vi "prepare_and_upload.vi"() -> ()   [LabVIEW 2016]
uses:
  <userlib>/LevyLab/Graph Utilities/graph_utilities.lvclass
  <userlib>/LevyLab/LV to ITX/Data/Data.lvclass
  <userlib>/LevyLab/postgreSQL-timescaleDB/Data.S3/Data.S3.lvclass
  <userlib>/LevyLab/postgreSQL-timescaleDB/Data.PG/Data.PGSQL.lvclass
  <userlib>/LevyLab/Graph Utilities/graph_utilities.lvclass/graph_utilities.ctl
  <userlib>/LevyLab/LV to ITX/Data/Data.lvclass/Data.ctl
  subvi/operationQueue/fft/fft_typedef.ctl
  subvi/operationQueue/derivative/derivative_typedef.ctl
  <userlib>/LevyLab/LV to ITX/Data/Typedefs/File Type--enum.ctl
  <userlib>/_OpenG.lib/file/file.llb/File Exists - Scalar__ogtk.vi
  <userlib>/_OpenG.lib/dictionary/dictionary.llb/Dictionary Update (by scalar value)__ogtk.vi
  <userlib>/LevyLab/XY Utilities/subVIs/Derivative (multiple).vi
  <userlib>/_OpenG.lib/file/file.llb/Build Path - File Names Array__ogtk.vi
  <userlib>/LevyLab/XY Utilities/xy_utilities.lvlib
  <userlib>/LevyLab/LV to ITX/Macros/Conversion.lvclass
panel:
  out "selected.local path":path
  out "generated tdms file path":path
  out "Intensity Graph":dbl[][](graph)
  out "Wavenames":string[](array[string])
  out "Notes":string
  out "Vertical Linecut":cluster{"Array":dbl[], "A x Vector":dbl[]}[](graph) caption="XY Graph"
  out "Horizontal Linecut":cluster{"Array":dbl[], "A x Vector":dbl[]}[](graph) caption="XY Graph"
  in  "# std deviations for\nhistogram width":dbl(slide)=1.4340101522842639 scale=0.0..5.0
  out "Histogram Graph":T1(graph)={"X Values"=[-4.260453721936876e-06, -4.186170219584622e-06, -4.111886717232367e-06, -4.037603214880112e-06, -3.9633197125278575e-06, -3.889036210175604e-06, -3.814752707823349e-06, -3.7404692054710943e-06, -3.6661857031188396e-06, -3.591902200766585e-06, -3.5176186984143303e-06, -3.4433351960620756e-06, -3.369051693709821e-06, -3.294768191357566e-06, -3.2204846890053115e-06, -3.1462011866530572e-06, -3.0719176843008025e-06, -2.9976341819485483e-06, -2.9233506795962936e-06, -2.849067177244039e-06, -2.774783674891784e-06, -2.7005001725395295e-06, -2.626216670187275e-06, -2.55193316783502e-06, -2.4776496654827654e-06, -2.4033661631305107e-06, -2.3290826607782565e-06, -2.2547991584260018e-06, -2.180515656073747e-06, -2.106232153721493e-06, -2.031948651369238e-06, -1.9576651490169834e-06, -1.8833816466647288e-06, -1.809098144312474e-06, -1.7348146419602196e-06, -1.6605311396079651e-06, -1.5862476372557104e-06, -1.5119641349034557e-06, -1.437680632551201e-06, -1.3633971301989466e-06, -1.289113627846692e-06, -1.2148301254944374e-06, -1.1405466231421827e-06, -1.066263120789928e-06, -9.919796184376733e-07, -9.176961160854188e-07, -8.434126137331644e-07, -7.691291113809097e-07, -6.94845609028655e-07, -6.205621066764003e-07, -5.462786043241458e-07, -4.7199510197189133e-07, -3.9771159961963664e-07, -3.2342809726738195e-07, -2.4914459491512726e-07, -1.7486109256287257e-07, -1.0057759021061788e-07, -2.6294087858363186e-08, 4.798941449389108e-08, 1.2227291684614535e-07, 1.9655641919840004e-07, 2.7083992155065473e-07, 3.451234239029094e-07, 4.194069262551641e-07, 4.936904286074188e-07, 5.679739309596735e-07, 6.422574333119282e-07, 7.165409356641829e-07, 7.908244380164376e-07, 8.651079403686918e-07, 9.393914427209461e-07, 1.0136749450732008e-06, 1.0879584474254555e-06, 1.1622419497777102e-06, 1.2365254521299649e-06, 1.3108089544822195e-06, 1.3850924568344742e-06, 1.459375959186729e-06, 1.5336594615389836e-06, 1.6079429638912379e-06, 1.6822264662434922e-06, 1.7565099685957468e-06, 1.8307934709480015e-06, 1.9050769733002562e-06, 1.979360475652511e-06, 2.0536439780047656e-06, 2.1279274803570203e-06, 2.202210982709275e-06, 2.2764944850615297e-06, 2.3507779874137844e-06, 2.4250614897660386e-06, 2.499344992118293e-06, 2.5736284944705476e-06, 2.6479119968228023e-06, 2.722195499175057e-06, 2.7964790015273117e-06, 2.8707625038795664e-06, 2.945046006231821e-06, 3.0193295085840757e-06, 3.09361301093633e-06], "Histogram: h(x)"=[55, 64, 64, 55, 89, 72, 77, 95, 93, 93, 89, 83, 103, 107, 94, 103, 104, 123, 108, 131, 122, 143, 132, 148, 168, 174, 204, 248, 183, 187, 243, 200, 217, 226, 238, 254, 185, 182, 212, 219, 221, 318, 385, 545, 593, 736, 735, 784, 778, 858, 957, 1241, 1705, 2411, 3715, 13259, 21719, 20305, 20447, 22279, 10136, 3576, 2142, 1564, 1112, 936, 844, 776, 734, 696, 601, 535, 390, 337, 334, 301, 271, 341, 294, 279, 254, 216, 170, 148, 122, 140, 100, 114, 127, 147, 102, 114, 129, 135, 110, 105, 90, 91, 93, 96]}
  in  "menu select":T2(tab)
  in  "Upload TDMS button":bool
  in  "View before uploading?":bool
  out "Converting Indicator":bool
  out "Uploading Indicator":bool
  in  "Populate Local Tree":bool
  in  "Local Tree":string(tree)
  in  "Populate Remote Tree":bool
  in  "local data directory":path=path "C:/bigdata/PPMS2/SA03008N.20190801/031_sg1_-1'1''5m_3AC=500m_bg=-14" caption="Path"
  out "Visualizing Indicator":bool
  out "TDMS load (ms)":u32
  out "data dimensions":i32[](array[numeric])
  in  "Remote Tree":string(tree)
  in  "path to aws credentials":path=path "C:/Users/phil/.aws/credentials"
  in  "aws bucket":string="levylab-data"
  out "generate TDMS (ms)":u32
  out "S3 upload (ms)":u32
  in  "connection info":T3
  in  "Operation Config":enum32{"derivative", "fft"}(tab)
  in  "derivative":T4={"derivative"="derivative", "Interval"=2.0, "Interval Units"=enum."Points", "Type"=enum."dy/dx vs x"}
  in  "Add Op":bool
  in  "Operations List":i32(listbox)
  in  "update":bool
  out "slicing\ntime":i32
  out "updating":bool
  in  "auto\nupdate":bool
  in  "trash can":i32(listbox)
  in  "OK":bool
  # "temporary things:"
  # "4"
  # "7"
  # "10"
  # "12"
  # "14"
  # "Settings"
  # "17"
  # "e.g. SA03008N.20190801"
  # "DON'T DOUBLE CLICK BIG FOLDERS"
  # ":)"
  # "not yet implemented"
  # "no settings"
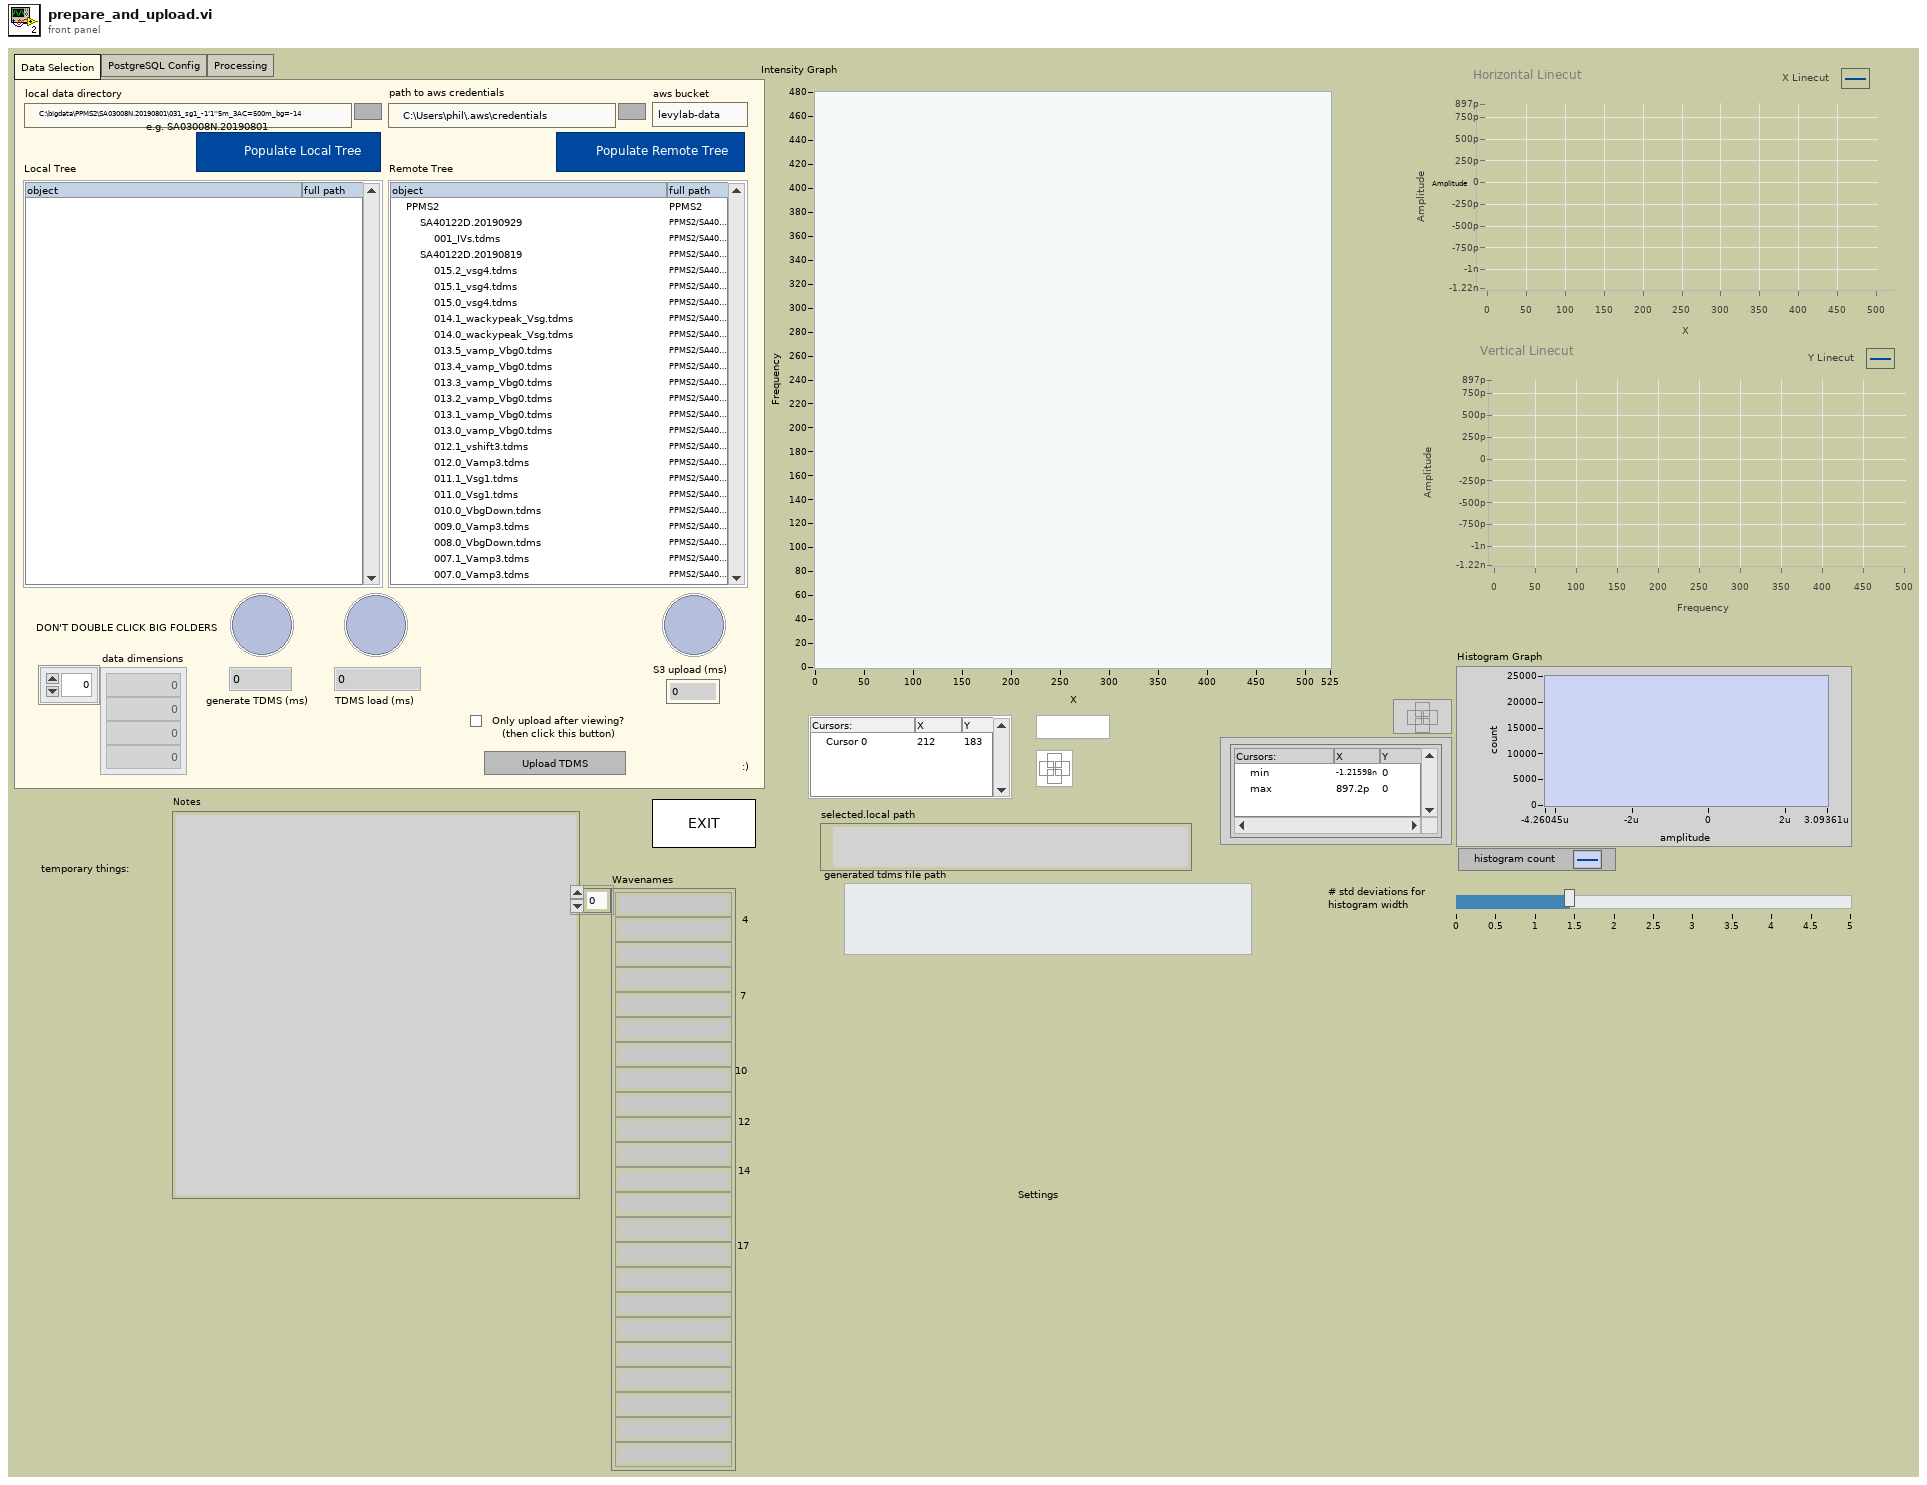
[diagram p1: front panel]
types:
  T1 = cluster{"X Values":dbl[], "Histogram: h(x)":i32[]}
  T2 = enum32{"Data Selection", "PostgreSQL Config", "Processing"}
  T3 = cluster{"host":string, "port":string, "user":string, "dbname":string, "password":string}
  T4 = cluster{"derivative":string, "Interval":dbl, "Interval Units":enum16{"Points", "Data"}, "Type":enum16{"dy/dx vs x", "dx/dy vs y"}}
  T5 = enum32{"Invalid", "Standard", "Closed", "Hidden", "Minimized", "Maximized"}
  T6 = enum32{"invalid app kind", "Development System", "Run Time System", "Student Edition", "Embedded LabVIEW", "Evaluation", "Custom"}
  T7 = typedef "fft_typedef.ctl" = cluster{"fft":string}
  T8 = typedef "derivative_typedef.ctl" = cluster{"derivative":string, "Interval":dbl, "Interval Units":enum16{"Points", "Data"}, "Type":enum16{"dy/dx vs x", "dx/dy vs y"}}
  T9 = typedef "Data.lvclass/File Type--enum.ctl" = enum16{"DAT", "ITX", "TDMS", "VI"}
  T10 = typedef "Dictionary Object RefNum__ogtk.ctl" = refnum<k1>
  T11 = cluster{"Core":cluster{"Current VI Reference":refnum<vi>, "Close Panel on Exit?":bool}, "active XY data":cluster{"All expt data":dbl[], "All expt data":dbl[]}[], "local data directory":path, "Data Save":refnum<class "Data.lvclass">, "graphs":refnum<class "graph_utilities.lvclass">[], "dictionary out":T10, "Operations List":refnum<vi>, "operations performed":string[], "Histogram Data":cluster{"X Values":dbl[], "Histogram: h(x)":i32[]}, "Histogram Graph":refnum<vi>, "wavenames":string[], "Data.S3":refnum<class "Data.S3.lvclass">, "data dimensions":i32[], "Data.PG in":refnum<class "Data.PGSQL.lvclass">, "selected":cluster{"local path":path, "\\ remote path":string, "/ remote path":string}, "generated tdms":path, "uploaded remote path":string}
  T12 = cluster{"local path":path, "\\ remote path":string, "/ remote path":string}
  T13 = cluster{"All expt data":dbl[], "All expt data":dbl[]}[]
  T14 = cluster{"Current VI Reference":refnum<vi>, "Close Panel on Exit?":bool}
  T15 = typedef "Data.lvclass/Dictionary--cluster.ctl" = cluster{"key":string, "value":variant}
  T16 = cluster{"concatenated string":string, "derivative":cluster{"derivative":string, "Interval":dbl, "Interval Units":enum16{"Points", "Data"}, "Type":enum16{"dy/dx vs x", "dx/dy vs y"}}}
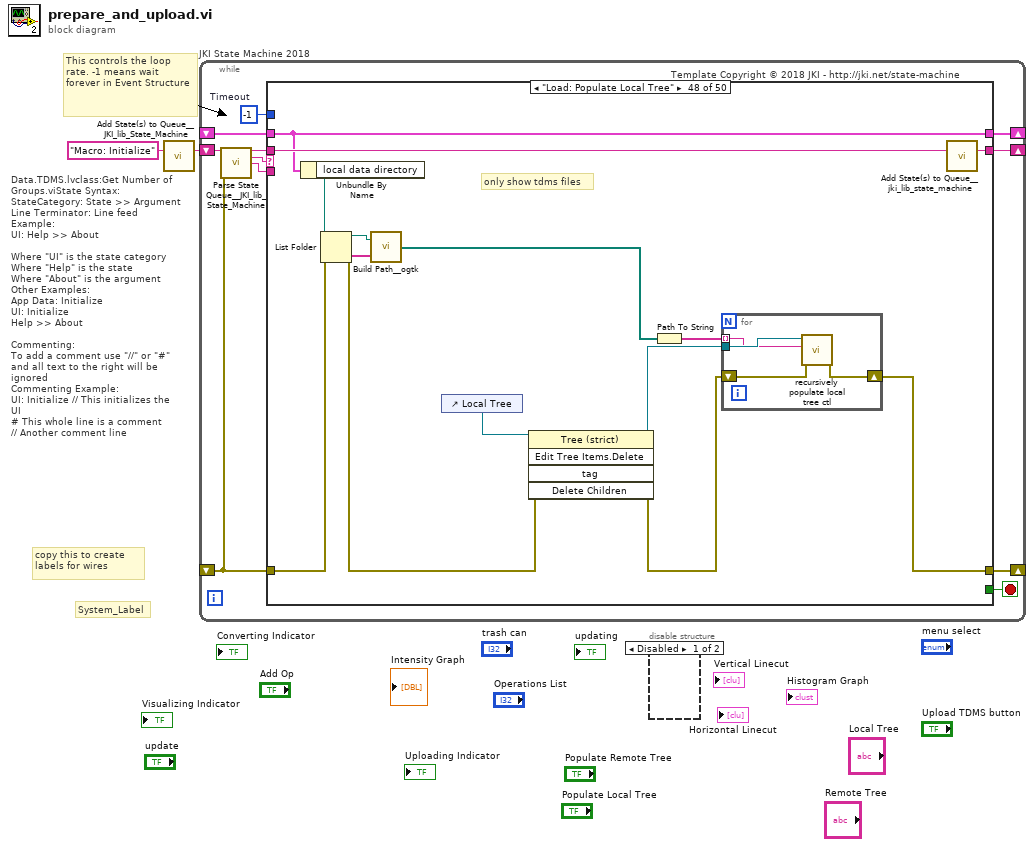
[diagram p0: block diagram]
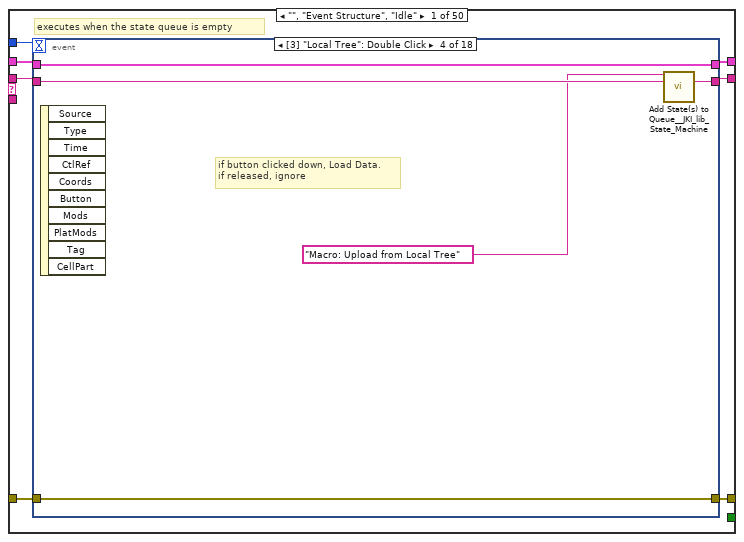
[diagram p3: hidden frame]
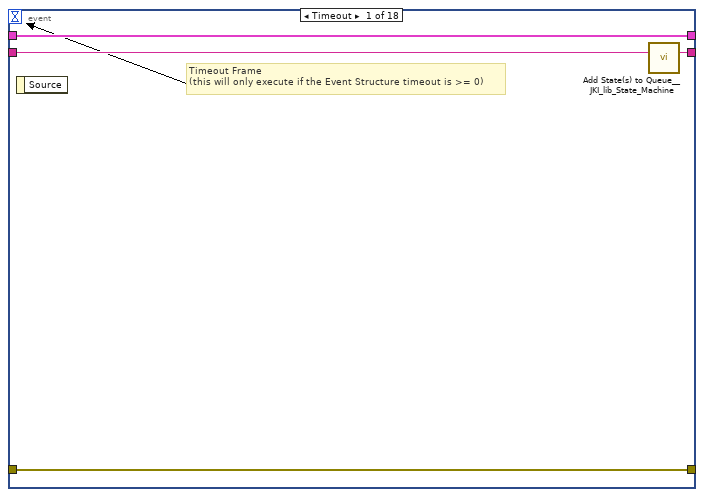
[diagram p4: hidden frame]
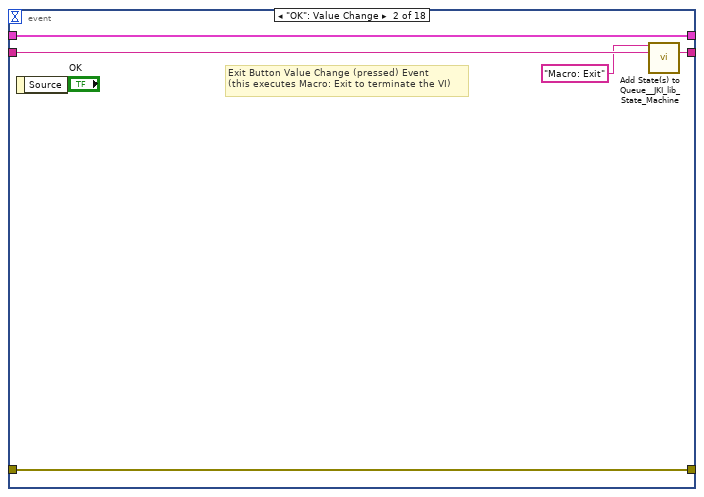
[diagram p5: hidden frame]
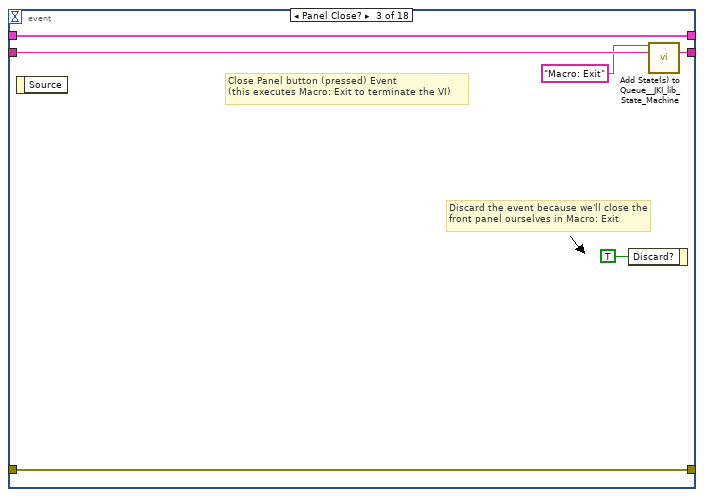
[diagram p6: hidden frame]
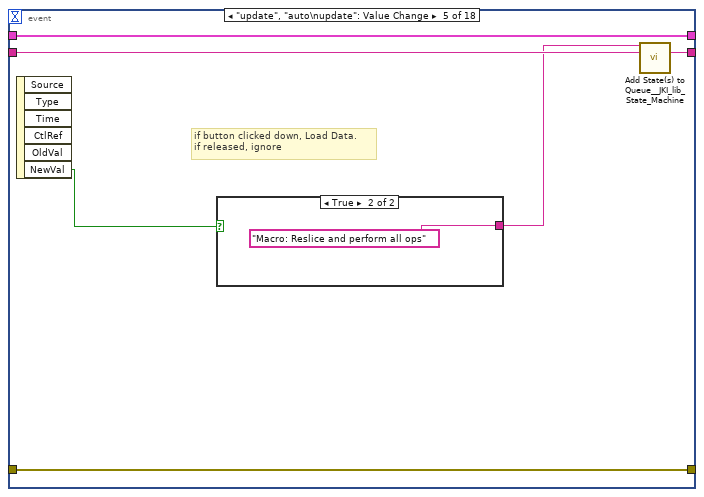
[diagram p7: hidden frame]
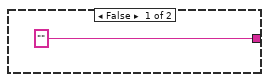
[diagram p8: hidden frame]
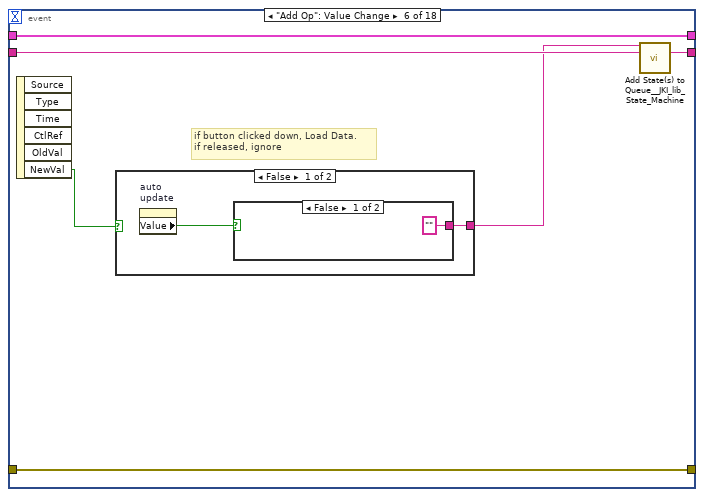
[diagram p9: hidden frame]
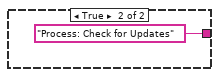
[diagram p10: hidden frame]
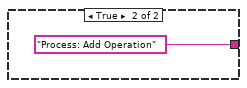
[diagram p11: hidden frame]
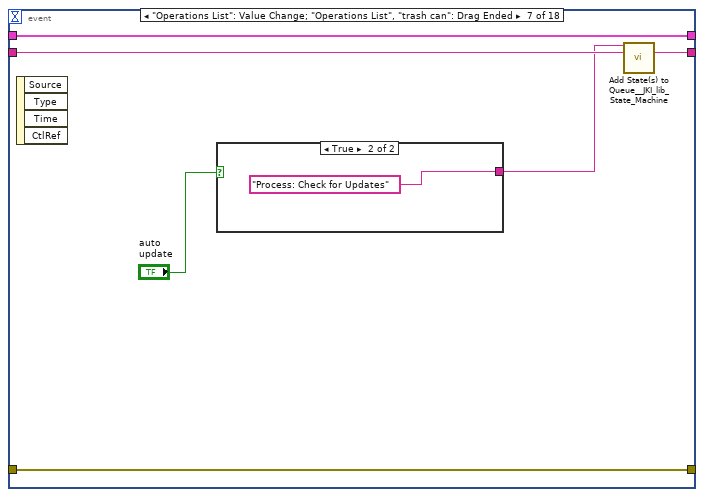
[diagram p12: hidden frame]
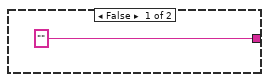
[diagram p13: hidden frame]
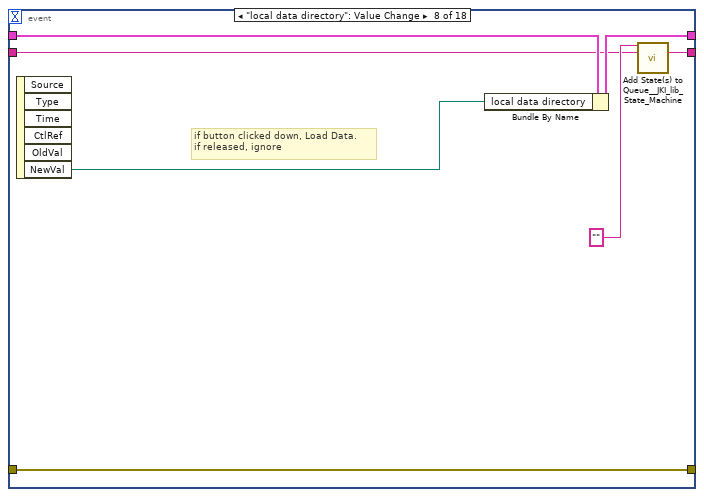
[diagram p14: hidden frame]
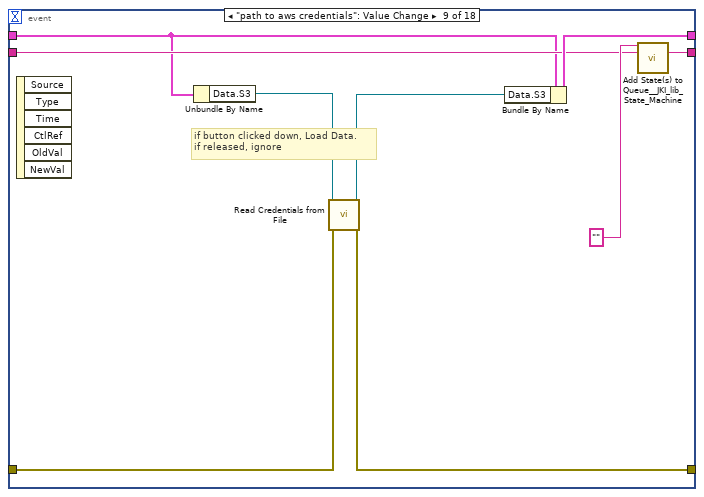
[diagram p15: hidden frame]
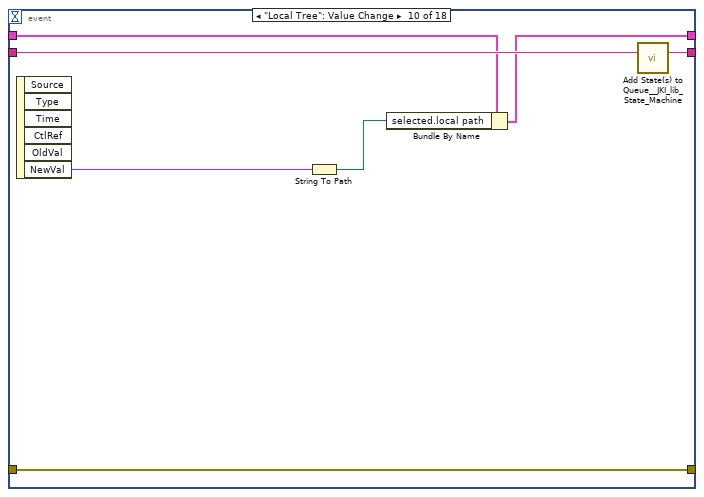
[diagram p16: hidden frame]
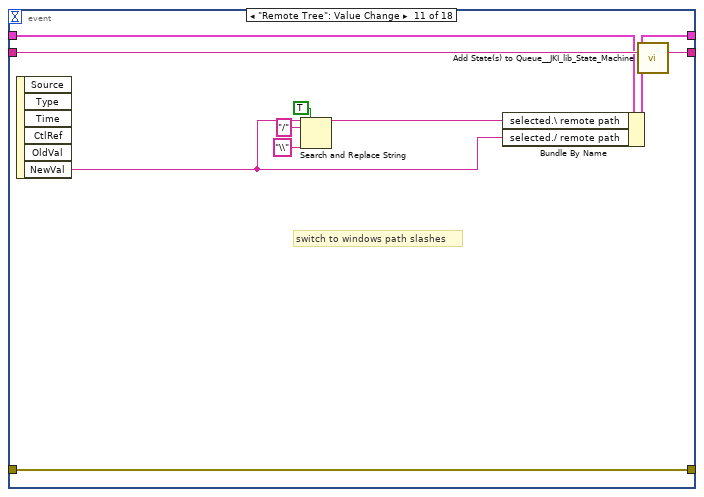
[diagram p17: hidden frame]
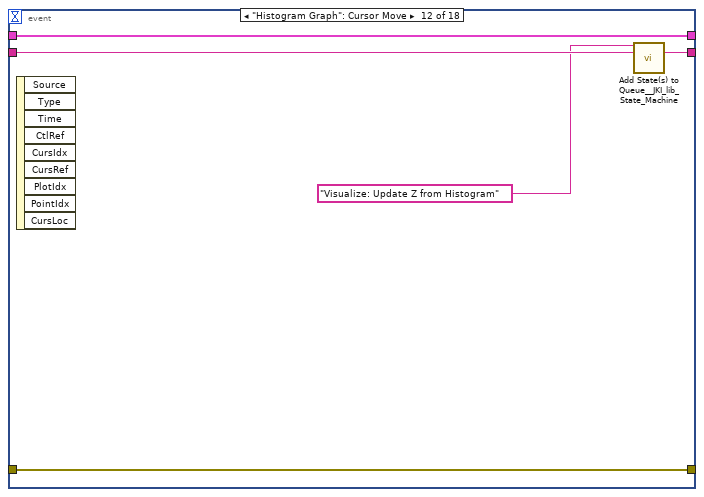
[diagram p18: hidden frame]
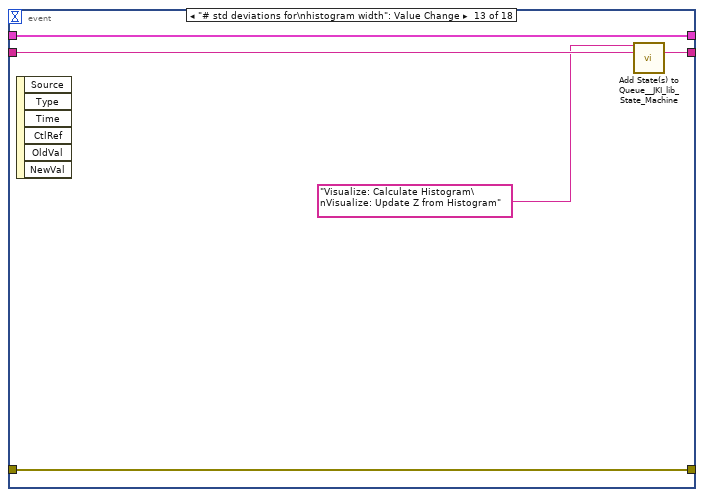
[diagram p19: hidden frame]
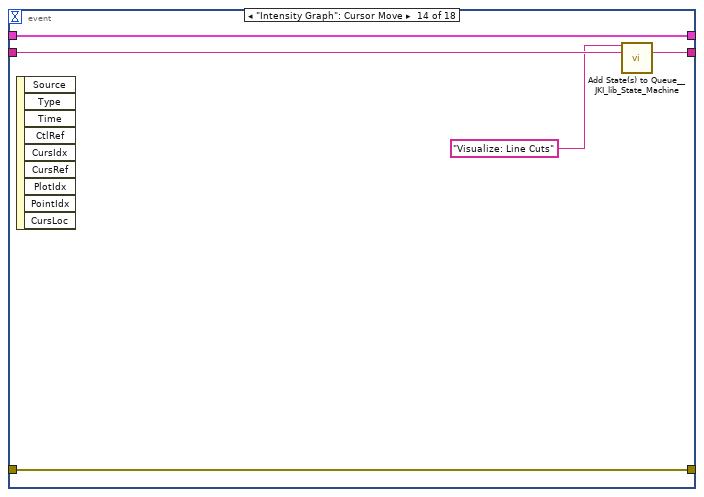
[diagram p20: hidden frame]
diagram:
  # "Data.TDMS.lvclass:Get Number of Groups.viState Syntax:\nStateCategory: State >> Argument\nLine Terminator: Line feed\nExample:\nUI: Help >> About\n\nWhere \"UI\" is the state category\nWhere \"Help\" is the state\nWhere \"About\" is the argument\nOther Examples:\nApp Data: Initialize\nUI: Initialize\nHelp >> About\n\nCommenting:\nTo add a comment use \"//\" or \"#\" and all text to the right will be ignored\nCommenting Example:\nUI: Initialize // This initializes the UI\n# This whole line is a comment\n// Another comment line"
  # "copy this to create labels for wires"
  # "This controls the loop rate. -1 means wait forever in Event Structure"
  # "System_Label"
  n1 = call <vilib>:"Add State(s) to Queue__JKI_lib_State_Machine.vi"("State(s) in (\"\")"="Macro: Initialize") -> ("States Out"=w2:string)  [unwired: 14 in]
  n2 = while "JKI State Machine 2018" {
    shift-right: [w6] -> _
    shift-left: _ -> [w3]
    shift-right: [w9] -> _
    shift-left: _ -> [w4]
    shift-right: [w8] -> _
    shift-left: w2 -> [w10]
    stop <- w7 stop-if-true
    w5 = -1  # Timeout
    # "Template Copyright © 2018 JKI - http://jki.net/state-machine"
    n3 = call <vilib>:"Parse State Queue__JKI_lib_State_Machine.vi"("State Queue"=w10, "Error In (no error)"=w4) -> ("Remaining States"=w12:string, "Current State"=w13:string, "Arguments"=w11:string)  [unwired: 11 in]
    n4 = case shown="\"Load: Populate Local Tree\"" w13 {
      selector: w13 -> [_ _ w149 _ _ _ _ _ _ _ _ _ _ _ _ _ _ _ _ _ _ _ _ _ _ _ _ _ _ _ _ _ _ _ _ _ _ _ _ _ _ _ _ _ _ _ _ _ _ _]
      tunnel: w12 -> [w20 w148 w153 w172 w178 w183 w187 w211 w237 w247 w251 w255 w261 w272 w341 w346 w356 w369 w374 w379 w384 w389 w394 w404 w408 w412 w416 w420 w424 w433 w467 w488 w492 w497 w501 w505 w523 w542 w549 w576 w613 w629 w644 w662 w676 w680 w709 w723 w731 w752]
      tunnel: w11 -> [_ _ _ _ _ _ _ _ _ _ _ _ w256 w266 _ _ _ _ _ _ _ _ _ _ _ _ _ _ _ _ _ _ _ _ _ _ _ _ _ _ _ _ _ _ _ _ _ _ _ _]
      tunnel: w3 -> [w18 w145 w151 w165 w175 w181 w184 _ w226 w242 w248 w253 w259 w268 w338 w343 w352 w366 w371 w376 w381 w386 w391 w401 w405 w409 w413 w417 w422 w427 w456 w486 w489 w494 w498 w502 w525 w543 w555 w579 w610 w621 w640 w660 w674 w677 w703 w721 w728 w734]
      tunnel: [w17 w146 w155 w169 errorcluster {"status"=FALSE, "code"=0, "source"=""} ("error out") w180 w185 w204 w212 w243 w249 w252 w257 w269 w339 w344 w353 w365 w370 w375 w380 w385 w390 w402 w406 w410 w414 w418 w421 w428 w449 w482 w490 w495 w499 w503 w529 w545 w557 w580 w611 w620 w632 w653 w666 w678 w705 w717 w729 w742] -> w9
      tunnel: w4 -> [w16 w146 w154 w169 w174 w180 w185 w205 w218 w244 w249 w252 w258 w270 w339 w344 w353 w365 w370 w375 w380 w385 w390 w402 w406 w410 w414 w418 w421 w429 w450 w477 w490 w495 w499 w503 w530 w545 w558 w580 w611 w622 w641 w654 w667 w678 w707 w711 w729 w742]
      tunnel: [w19 w147 w152 w171 w177 w182 w186 w210 w236 w246 w250 w254 w260 w271 w340 w345 w355 w368 w373 w378 w383 w388 w393 w403 w407 w411 w415 w419 w423 w432 w466 w487 w491 w496 w500 w504 w523 w541 w549 w576 w612 w628 w643 w661 w675 w679 w708 w722 w730 w751] -> w8
      tunnel: [_ _ _ _ _ TRUE _ _ _ _ _ _ _ _ _ _ _ _ _ _ _ _ _ _ _ _ _ _ _ _ _ _ _ _ _ _ _ _ _ _ _ _ _ _ _ _ _ _ _ _] -> w7
      tunnel: [w15 w145 w151 w170 w175 w181 w184 w209 w235 w242 w248 w253 w259 w268 w338 w343 w352 w366 w371 w376 w381 w386 w391 w401 w405 w409 w413 w417 w422 w426 w457 w486 w489 w494 w498 w502 w524 w543 w555 w578 w610 w621 w640 w660 w674 w677 w702 w721 w728 w733] -> w6
      tunnel: w5 -> [w14 _ _ _ _ _ _ _ _ _ _ _ _ _ _ _ _ _ _ _ _ _ _ _ _ _ _ _ _ _ _ _ _ _ _ _ _ _ _ _ _ _ _ _ _ _ _ _ _ _]
      frame "", "Event Structure", "Idle" {
        # "executes when the state queue is empty"
        n5 = event shown="[3] \"Local Tree\": Double Click" {
          selector: _ -> [_ _ _ _ _ _ _ _ _ _ _ _ _ _ _ _ _ _]
          dyn-events: _ -> [_ _ _ _ _ _ _ _ _ _ _ _ _ _ _ _ _ _]
          timeout: w14 -> [_ _ _ _ _ _ _ _ _ _ _ _ _ _ _ _ _ _]
          tunnel: w20 -> [w24 w29 w35 w37 w43 w51 w64 w69 w80 w88 w98 w103 w108 w112 w118 w126 w134 w141]
          tunnel: [w23 w28 w34 w38 w44 w52 w63 w70 w81 w89 w99 w102 w107 w113 w119 w127 w135 w142] -> w19
          tunnel: w18 -> [w21 w26 w32 w40 w46 w54 w60 w73 w79 w87 w97 w105 w110 w115 w121 w129 w137 w144]
          tunnel: [w22 w27 w33 w39 w45 w53 w65 w74 w75 w90 w100 w104 w109 w114 w120 w128 w136 w143] -> w17
          tunnel: w16 -> [w22 w27 w33 w39 w45 w53 w65 w74 w76 w90 w100 w104 w109 w114 w120 w128 w136 w143]
          tunnel: [w21 w26 w32 w40 w46 w54 w60 w72 w83 w86 w96 w105 w110 w115 w121 w129 w137 w144] -> w15
          event Timeout {
            # "Timeout Frame\n(this will only execute if the Event Structure timeout is >= 0)"
            n6 = event-data() -> ()  [unwired: 1 in, 1 out]
            n7 = call <vilib>:"Add State(s) to Queue__JKI_lib_State_Machine.vi"("State(s) in (\"\")"=w24) -> ("States Out"=w23:string)  [unwired: 14 in]
          }
          event "OK": Value Change {
            # "Exit Button Value Change (pressed) Event\n(this executes Macro: Exit to terminate the VI)"
            n8 = event-data() -> ()  [unwired: 1 in, 1 out]
            n9 = call <vilib>:"Add State(s) to Queue__JKI_lib_State_Machine.vi"("State(s) in Front (\"\")"="Macro: Exit", "State(s) in (\"\")"=w29) -> ("States Out"=w28:string)  [unwired: 13 in]
          }
          event Panel Close? {
            # "Discard the event because we'll close the front panel ourselves in Macro: Exit"
            # "Close Panel button (pressed) Event\n(this executes Macro: Exit to terminate the VI)"
            n10 = event-data() -> ()  [unwired: 1 in, 1 out]
            n11 = event-data("Discard?"=TRUE) -> ()  [unwired: 1 in, 1 out]
            n12 = call <vilib>:"Add State(s) to Queue__JKI_lib_State_Machine.vi"("State(s) in Front (\"\")"="Macro: Exit", "State(s) in (\"\")"=w35) -> ("States Out"=w34:string)  [unwired: 13 in]
          }
          event "Local Tree": Double Click {
            # "if button clicked down, Load Data.\nif released, ignore"
            n13 = event-data() -> ()  [unwired: 1 in, 10 out]
            n14 = call <vilib>:"Add State(s) to Queue__JKI_lib_State_Machine.vi"("State(s) in Front (\"\")"="Macro: Upload from Local Tree", "State(s) in (\"\")"=w37) -> ("States Out"=w38:string)  [unwired: 13 in]
          }
          event "update", "auto\nupdate": Value Change {
            # "if button clicked down, Load Data.\nif released, ignore"
            n15 = event-data() -> ("NewVal"=w42:bool)  [unwired: 1 in, 5 out]
            n16 = case shown="True" w42 {
              tunnel: ["" "Macro: Reslice and perform all ops"] -> w41
              frame False {
              }
              frame True {
              }
            }
            n17 = call <vilib>:"Add State(s) to Queue__JKI_lib_State_Machine.vi"("State(s) in Front (\"\")"=w41, "State(s) in (\"\")"=w43) -> ("States Out"=w44:string)  [unwired: 13 in]
          }
          event "Add Op": Value Change {
            # "if button clicked down, Load Data.\nif released, ignore"
            n18 = event-data() -> ("NewVal"=w50:bool)  [unwired: 1 in, 5 out]
            n19 = case shown="False" w50 {
              tunnel: [w56 "Process: Add Operation"] -> w49
              frame False {
                n20 = property on="auto\nupdate" class="Bool (strict)"() -> ("Value"=w55:bool)  [unwired: 2 in, 2 out]
                n21 = case shown="False" w55 {
                  tunnel: ["" "Process: Check for Updates"] -> w56
                  frame False {
                  }
                  frame True {
                  }
                }
              }
              frame True {
              }
            }
            n22 = call <vilib>:"Add State(s) to Queue__JKI_lib_State_Machine.vi"("State(s) in Front (\"\")"=w49, "State(s) in (\"\")"=w51) -> ("States Out"=w52:string)  [unwired: 13 in]
          }
          event "Operations List": Value Change; "Operations List", "trash can": Drag Ended {
            n23 = event-data() -> ()  [unwired: 1 in, 4 out]
            n24 = case shown="True" "auto\nupdate" {
              tunnel: ["" "Process: Check for Updates"] -> w62
              frame False {
              }
              frame True {
              }
            }
            n25 = call <vilib>:"Add State(s) to Queue__JKI_lib_State_Machine.vi"("State(s) in Front (\"\")"=w62, "State(s) in (\"\")"=w64) -> ("States Out"=w63:string)  [unwired: 13 in]
          }
          event "local data directory": Value Change {
            # "if button clicked down, Load Data.\nif released, ignore"
            n26 = event-data() -> ("NewVal"=w68:path)  [unwired: 1 in, 5 out]
            n27 = Bundle By Name(cluster=w73, "local data directory"=w68) -> (w72:T11)
            n28 = call <vilib>:"Add State(s) to Queue__JKI_lib_State_Machine.vi"("State(s) in Front (\"\")"="" ("State(s) in Front (\"\")"), "State(s) in (\"\")"=w69) -> ("States Out"=w70:string)  [unwired: 13 in]
          }
          event "path to aws credentials": Value Change {
            # "if button clicked down, Load Data.\nif released, ignore"
            n29 = event-data() -> ()  [unwired: 1 in, 6 out]
            n30 = Unbundle By Name(w79) -> ("Data.S3"=w78:refnum<class "Data.S3.lvclass">)
            n31 = call <userlib>:"Read Credentials from File.vi"("error in (no error)"=w76, "Data.S3"=w78) -> ("error out"=w75:errorcluster, "Data.S3 out"=w77:refnum<class "Data.S3.lvclass">)  [unwired: 8 in]
            n32 = Bundle By Name(cluster=w79, "Data.S3"=w77) -> (w83:T11)
            n33 = call <vilib>:"Add State(s) to Queue__JKI_lib_State_Machine.vi"("State(s) in Front (\"\")"="" ("State(s) in Front (\"\")"), "State(s) in (\"\")"=w80) -> ("States Out"=w81:string)  [unwired: 13 in]
          }
          event "Local Tree": Value Change {
            n34 = event-data() -> ("NewVal"=w84:string)  [unwired: 1 in, 5 out]
            n35 = String To Path(string=w84) -> (path=w85:path)
            n36 = Bundle By Name(cluster=w87, "selected.local path"=w85) -> (w86:T11)
            n37 = call <vilib>:"Add State(s) to Queue__JKI_lib_State_Machine.vi"("State(s) in (\"\")"=w88) -> ("States Out"=w89:string)  [unwired: 14 in]
          }
          event "Remote Tree": Value Change {
            # "switch to windows path slashes"
            n38 = event-data() -> ("NewVal"=w92:string)  [unwired: 1 in, 5 out]
            n39 = Search and Replace String(replace all?=TRUE ("replace all? (F)"), input string=w92, search string="/", replace string="\\" ("replace string (\"\")")) -> (result string=w93:string)  [unwired: 4 in, 3 out]
            n40 = Bundle By Name(cluster=w97, "selected.\\ remote path"=w93, "selected./ remote path"=w92) -> (w96:T11)
            n41 = call <vilib>:"Add State(s) to Queue__JKI_lib_State_Machine.vi"("State(s) in (\"\")"=w98) -> ("States Out"=w99:string)  [unwired: 14 in]
          }
          event "Histogram Graph": Cursor Move {
            n42 = event-data() -> ()  [unwired: 1 in, 9 out]
            n43 = call <vilib>:"Add State(s) to Queue__JKI_lib_State_Machine.vi"("State(s) in Front (\"\")"="Visualize: Update Z from Histogram" ("State(s) in Front (\"\")"), "State(s) in (\"\")"=w103) -> ("States Out"=w102:string)  [unwired: 13 in]
          }
          event "# std deviations for\nhistogram width": Value Change {
            n44 = event-data() -> ()  [unwired: 1 in, 6 out]
            n45 = call <vilib>:"Add State(s) to Queue__JKI_lib_State_Machine.vi"("State(s) in Front (\"\")"="Visualize: Calculate Histogram\nVisualize: Update Z from Histogram" ("State(s) in Front (\"\")"), "State(s) in (\"\")"=w108) -> ("States Out"=w107:string)  [unwired: 13 in]
          }
          event "Intensity Graph": Cursor Move {
            n46 = event-data() -> ()  [unwired: 1 in, 9 out]
            n47 = call <vilib>:"Add State(s) to Queue__JKI_lib_State_Machine.vi"("State(s) in Front (\"\")"="Visualize: Line Cuts" ("State(s) in Front (\"\")"), "State(s) in (\"\")"=w112) -> ("States Out"=w113:string)  [unwired: 13 in]
          }
          event "Populate Remote Tree": Value Change {
            n48 = event-data() -> ("NewVal"=w116:bool)  [unwired: 1 in, 5 out]
            n49 = case shown="True" w116 {
              tunnel: ["" "Macro: Populate Remote Tree" ("State(s) in Front (\"\")")] -> w117
              frame False {
              }
              frame True {
              }
            }
            n50 = call <vilib>:"Add State(s) to Queue__JKI_lib_State_Machine.vi"("State(s) in Front (\"\")"=w117, "State(s) in (\"\")"=w118) -> ("States Out"=w119:string)  [unwired: 13 in]
          }
          event "Populate Local Tree": Value Change {
            n51 = event-data() -> ("NewVal"=w124:bool)  [unwired: 1 in, 5 out]
            n52 = case shown="True" w124 {
              tunnel: ["" "Macro: Populate Local Tree" ("State(s) in Front (\"\")")] -> w125
              frame False {
              }
              frame True {
              }
            }
            n53 = call <vilib>:"Add State(s) to Queue__JKI_lib_State_Machine.vi"("State(s) in Front (\"\")"=w125, "State(s) in (\"\")"=w126) -> ("States Out"=w127:string)  [unwired: 13 in]
          }
          event "Upload TDMS button": Value Change {
            n54 = event-data() -> ("NewVal"=w132:bool)  [unwired: 1 in, 5 out]
            n55 = case shown="True" w132 {
              tunnel: ["" "Macro: Upload to AWS" ("State(s) in Front (\"\")")] -> w133
              frame False {
              }
              frame True {
              }
            }
            n56 = call <vilib>:"Add State(s) to Queue__JKI_lib_State_Machine.vi"("State(s) in Front (\"\")"=w133, "State(s) in (\"\")"=w134) -> ("States Out"=w135:string)  [unwired: 13 in]
          }
          event "Remote Tree": Double Click {
            # "do nothing"
            n57 = event-data() -> ()  [unwired: 1 in, 10 out]
            n58 = call <vilib>:"Add State(s) to Queue__JKI_lib_State_Machine.vi"("State(s) in Front (\"\")"="" ("State(s) in Front (\"\")"), "State(s) in (\"\")"=w141) -> ("States Out"=w142:string)  [unwired: 13 in]
          }
        }
      }
      frame "---------- Core ----------" {
        # "Do not put any code in this frame.\n(it is a separator no-op)"
        n59 = call <vilib>:"Add State(s) to Queue__jki_lib_state_machine.vi"("State(s) in (\"\")"=w148) -> ("States Out"=w147:string)  [unwired: 14 in]
      }
      frame Default {
        w158 = 42 items=["No error", "Argument error", "Memory is full", "Out of zone", "End of file", "File already open", "Generic file I/O error", "File not found", "File permission error", "Disk is full", "Duplicate path", "Too many files open", "System feature not enabled", "Resource file not found", "Cannot add resource", "Resource not found", "Image not found", "Image memory error", "Pen does not exist", "Config type invalid", "Config token not found", "Config parse error", "Config memory error", "Bad external code format", "Bad external code offset", "External code not present", "Null window", "Destroy window error", "Null menu", "Print aborted", "Bad print record", "Print driver error", "Windows error during printing", "Memory error during printing", "Print dialog error", "Generic print error", "Invalid device refnum", "Device not found", "Device parameter error", "Device unit error", "Cannot open device", "Device call aborted", "Generic error", "Cancelled by user", "Object ID too low", "Object ID too high", "Object not in heap", "Unknown heap", "Unknown object (invalid DefProc)", "Unknown object (DefProc not in table)", "Message out of range", "Invalid (null) method", "Unknown message", "Manager call not supported", "Bad address", "Network operation in progress", "Network operation timed out", "Connection is busy", "Network attribute not supported", "Network error", "Address in use", "System out of memory", "Connection aborted", "Connection refused", "Not connected", "Already connected", "Connection closed", "Initialization error (interapplication manager)", "Bad occurrence", "Wait on unbound occurrence handler", "Occurrence queue overflow", "Datalog type conflict", "Unused", "Unrecognized type (interapplication manager)", "Memory corrupt", "Failed to make temporary DLL", "Old CIN version", "Drag socket not found", "Failed to load drop-object", "Failed to register OLE object", "Failed to release OLE object", "Format specifier type mismatch", "Unknown format specifier", "Too few format specifiers", "Too many format specifiers", "Scan failed", "Newer CIN version", "Error converting to variant", "Runtime menu error", "Password tampered", "Variant attribute not found", "Incompatible variant data type", "Event data is not available", "Event Store is not present", "Occurrence is not found", "Event Queue is not created", "Event info is not available", "Refnum passed is NULL", "Error retrieving Class GUID", "Error retrieving CoClass GUID", "Error retrieving TypeLib GUID.", "Bad built application magic bytes.", "Specific driver is different from the specific driver associated with the Logical Name.", "There is no session opened to the class driver.", "Max Error", "MAX - Error with config objects", "MAX - Error loading configuration", "MAX - Group not supported"]
        # "Current State"
        # "Do not delete, rename, or modify this frame.\n(this is used to capture unhandled states and typos)"
        # "Handle mistyped state name (developer tool)"
        n60 = Format Into String(format string="Software Exception: Unhandled State \"%s\"." ("message"), error in=w154, w149) -> (resulting string=w157:string, error out=w156:errorcluster)  [unwired: 1 in]
        n61 = call <vilib>:"Error Cluster From Error Code.vi"("show call chain? (False)"=TRUE, "error in (no error)"=w156, "error message (\"\")"=w157, "error code (0)"=w158) -> ("error out"=w155:errorcluster)  [unwired: 5 in]
        n62 = call <vilib>:"Add State(s) to Queue__jki_lib_state_machine.vi"("State(s) in (\"\")"=w153) -> ("States Out"=w152:string)  [unwired: 14 in]
      }
      frame "Initialize Core Data" {
        # "Do not delete, rename, or modify this frame.\n(this is used to determine panel behavior on exit)"
        # "originally closed?"
        # "exe?"
        # "If panel starts closed or is an EXE, then close it when we exit"
        n63 = property class="VI"() -> ("FP.State"=w162:T5)  [unwired: 2 in, 2 out]
        n64 = property class="App"() -> ("App.Kind"=w168:T6)  [unwired: 2 in, 2 out]
        n65 = control-ref of="Current VI Reference"() -> (w163:refnum<vi>)
        n66 = Equal?(x=w162, y=T5."Closed" ("Front Panel Window:State")) -> (x = y?=w160:bool)
        n67 = Equal?(x=w168, y=T6."Run Time System" ("Application:Kind")) -> (x = y?=w166:bool)
        n68 = Or(x=w160, y=w166) -> (x .or. y?=w164:bool)
        n69 = Bundle By Name(cluster=w165, "Core.Current VI Reference"=w163, "Core.Close Panel on Exit?"=w164) -> (w170:T11)
        n70 = call <vilib>:"Add State(s) to Queue__jki_lib_state_machine.vi"("State(s) in (\"\")"=w172) -> ("States Out"=w171:string)  [unwired: 14 in]
      }
      frame "Error Handler" {
        # "Unhandled Error -- Display it"
        # "Handle any errors here.\nYou can also output any states to clean-up after errors occur"
        # "Clear error"
        n71 = call <vilib>:"General Error Handler.vi"("error in (no error)"=w174) -> ()  [unwired: 10 in, 5 out]
        n72 = call <vilib>:"Add State(s) to Queue__jki_lib_state_machine.vi"("State(s) in Front (\"\")"="/* Post Error States", "State(s) in (\"\")"=w178) -> ("States Out"=w177:string)  [unwired: 13 in]
      }
      frame "Exit" {
        # "Do not put any code in this frame.\n(No errors that occur here will be handled.)"
        n73 = call <vilib>:"Add State(s) to Queue__jki_lib_state_machine.vi"("State(s) in (\"\")"=w183) -> ("States Out"=w182:string)  [unwired: 14 in]
      }
      frame "---------- Data ----------" {
        # "Do not put any code in this frame.\n(It is a separator no-op. You can make a copy of this frame to create a new Data frame)"
        n74 = call <vilib>:"Add State(s) to Queue__jki_lib_state_machine.vi"("State(s) in (\"\")"=w187) -> ("States Out"=w186:string)  [unwired: 14 in]
      }
      frame "Data: Initialize" {
        w189 = ""  # uploaded remote path
        w190 = path ""  # generated tdms
        w191 = T12 {"local path"=path "", "\\ remote path"="", "/ remote path"=""}  # selected
        w192 = i32[] []  # data dimensions
        w193 = refnum<class "Data.S3.lvclass"> refnum  # Data.S3
        w194 = string[] []  # wavenames
        w198 = T1 {"X Values"=[], "Histogram: h(x)"=[]}  # Histogram Data
        w199 = string[] []  # operations performed
        w201 = T13 []  # active XY data
        w200 = string[] [] ("Strings []")
        w207 = refnum<class "graph_utilities.lvclass">[] []  # graphs
        w208 = T14 {"Current VI Reference"=refnum, "Close Panel on Exit?"=FALSE}  # Core
        # "# groups in tdms\n    (i.e. # original itx files)\n# channels (time, AIN, AON,\n# points per channel\n    (except the channels\n     that only store 1)"
        # "do not delete - used by framework"
        # "Data names and types of shift register data are defined by this bundle."
        # "Initialize the shift-register data, here.\n(data names are defined by what you wire into the bundle function)"
        n75 = call <userlib>:"Dictionary Create__ogtk.vi"("error in (no error)"=w205) -> ("error out"=w204:errorcluster, "dictionary out"=w206:T10)  [unwired: 9 in]
        n76 = control-ref of="Operations List"() -> (w202:refnum<vi>)
        n77 = property on="trash can" class="LstBox (strict)"("Item Names"=w200) -> ()  [unwired: 2 in, 2 out]
        n78 = property class="LstBox (strict)"(reference=w202, "Item Names"=w200) -> (reference out=w203:refnum<vi>)  [unwired: 1 in, 1 out]
        n79 = control-ref of="Histogram Graph"() -> (w197:refnum<vi>)
        n80 = Bundle("Core"=w208, "active XY data"=w201, "local data directory"="local data directory", "Data Save"=refnum<class "Data.lvclass"> refnum, "graphs"=w207, "dictionary out"=w206, "Operations List"=w203, "operations performed"=w199, "Histogram Data"=w198, "Histogram Graph"=w197, "wavenames"=w194, "Data.S3"=w193, "data dimensions"=w192, "Data.PG in"=refnum<class "Data.PGSQL.lvclass"> refnum, "selected"=w191, "generated tdms"=w190, "uploaded remote path"=w189) -> (w209:T11)  [unwired: 1 in]
        n81 = call <vilib>:"Add State(s) to Queue__jki_lib_state_machine.vi"("State(s) in (\"\")"=w211) -> ("States Out"=w210:string)  [unwired: 14 in]
      }
      frame "Data: Initialize Graph References" {
        # "clear graph"
        # "need to somehow set credentials and bucket"
        n82 = control-ref of="Intensity Graph"() -> (w220:refnum<vi>)
        n83 = invoke on="Remote Tree" class="Tree (strict)" method="Edit Tree Items.Delete"(error in=w218) -> (error out=w217:errorcluster)  [unwired: 4 in, 4 out]
        n84 = control-ref of="Vertical Linecut"() -> (w229:refnum<vi>)
        n85 = Unbundle By Name(w226) -> ("Data.S3"=w225:refnum<class "Data.S3.lvclass">)
        n86 = property class="IntGraph (strict)"(reference=w220, "Value"=dbl[][] []) -> (reference out=w219:refnum<vi>)  [unwired: 1 in, 1 out]
        n87 = invoke on="Local Tree" class="Tree (strict)" method="Edit Tree Items.Delete"(error in=w217) -> (error out=w216:errorcluster)  [unwired: 4 in, 4 out]
        n88 = call-poly <userlib>:"File Exists__ogtk.vi"("file path"="path to aws credentials") -> ("exists"=w214:bool)  [unwired: 6 in, 1 out]
        n89 = control-ref of="Horizontal Linecut"() -> (w230:refnum<vi>)
        n90 = case shown="True" w214 {
          tunnel: w225 -> [w238 w241]
          tunnel: [w238 w240] -> w222
          tunnel: "path to aws credentials" -> [_ w239]
          frame False {
          }
          frame True {
            n91 = call <userlib>:"Read Credentials from File.vi"("path to aws credentials"=w239, "Data.S3"=w241) -> ("Data.S3 out"=w240:refnum<class "Data.S3.lvclass">)  [unwired: 8 in, 1 out]
          }
        }
        n92 = call <userlib>:"Set Bucket.vi"("Bucket name"="aws bucket", "Data.S3"=w222) -> ("Data.S3"=w224:refnum<class "Data.S3.lvclass">)  [unwired: 8 in, 1 out]
        n93 = call <userlib>:"Write Intensity Graph ref.vi"("error in (no error)"=w216, "Intensity Graph (Control)"=w219, "Intensity Graph"=w219) -> ("error out"=w233:errorcluster, "graph_utilities out"=w228:refnum<class "graph_utilities.lvclass">)  [unwired: 7 in]
        n94 = call <userlib>:"Write XY Graph ref.vi"("error in (no error)"=w233, "XY Graph"=w229, "graph_utilities in"=w228) -> ("error out"=w232:errorcluster, "graph_utilities out"=w227:refnum<class "graph_utilities.lvclass">)  [unwired: 7 in]
        n95 = call <userlib>:"Write XY Graph ref.vi"("error in (no error)"=w232, "XY Graph"=w230, "graph_utilities in"=w228) -> ("error out"=w212:errorcluster, "graph_utilities out"=w231:refnum<class "graph_utilities.lvclass">)  [unwired: 7 in]
        n96 = Build Array(w228, w227, w231) -> (w234:refnum<class "graph_utilities.lvclass">[])
        n97 = property on="Local Tree" class="Tree (strict)"(error in=w212, "Value"=" " ("Local Tree")) -> ()  [unwired: 1 in, 2 out]
        n98 = Bundle By Name(cluster=w226, "graphs"=w234, "Data.S3"=w224) -> (w235:T11)
        n99 = call <vilib>:"Add State(s) to Queue__jki_lib_state_machine.vi"("State(s) in (\"\")"=w237) -> ("States Out"=w236:string)  [unwired: 14 in]
      }
      frame "Data: Cleanup" {
        # "Cleanup any data and references, here.\n(this is called automatically, by the Macro: Exit)"
        n100 = Unbundle By Name(w242) -> ("Core.Current VI Reference"=w245:refnum<vi>)
        n101 = Close Reference(reference=w245, error in (no error)=w244) -> (error out=w243:errorcluster)
        n102 = call <vilib>:"Add State(s) to Queue__jki_lib_state_machine.vi"("State(s) in (\"\")"=w247) -> ("States Out"=w246:string)  [unwired: 14 in]
      }
      frame "---------- UI ----------" {
        # "Do not put any code in this frame.\n(It is a separator no-op. You can make a copy of this frame to create a new UI frame)"
        n103 = call <vilib>:"Add State(s) to Queue__jki_lib_state_machine.vi"("State(s) in (\"\")"=w251) -> ("States Out"=w250:string)  [unwired: 14 in]
      }
      frame "UI: Initialize" {
        # "Initialize the User Interface, here.\n(this is called automatically, by the Macro: Init)"
        n104 = call <vilib>:"Add State(s) to Queue__jki_lib_state_machine.vi"("State(s) in (\"\")"=w255) -> ("States Out"=w254:string)  [unwired: 14 in]
      }
      frame "UI: Cursor Set" {
        # "Argument"
        # "Set and Unset Cursor Busy.\n(Usage: \"UI: Cursor Set >> Busy|Idle\")"
        n105 = case shown="\"Idle\", Default" w256 {
          tunnel: w258 -> [w263 w265]
          tunnel: [w262 w264] -> w257
          frame "Idle", Default {
            n106 = call <vilib>:"Unset Busy.vi"("error in (no error)"=w263) -> ("error out"=w262:errorcluster)  [unwired: 10 in]
          }
          frame "Busy" {
            n107 = call <vilib>:"Set Busy.vi"("error in (no error)"=w265) -> ("error out"=w264:errorcluster)  [unwired: 9 in, 1 out]
          }
        }
        n108 = call <vilib>:"Add State(s) to Queue__jki_lib_state_machine.vi"("State(s) in (\"\")"=w261) -> ("States Out"=w260:string)  [unwired: 14 in]
      }
      frame "UI: Front Panel State" {
        # "Argument"
        # "Set Front Panel Open or Closed\n(Usage: \"UI: Front Panel State >> Open|Close\")"
        n109 = Unbundle By Name(w268) -> ("Core.Current VI Reference"=w267:refnum<vi>)
        n110 = case shown="\"Minimize\", \"Minimized\"" w266 {
          tunnel: w270 -> [w278 w293 w304 w317 w330]
          tunnel: [w280 w294 w306 w319 w332] -> w269
          tunnel: w267 -> [w279 w291 w305 w318 w331]
          frame "Open", "Standard", Default {
            w273 = T5."Standard" ("State")
            n111 = property class="VI"(reference=w279, error in=w278) -> (reference out=w276:refnum<vi>, error out=w277:errorcluster, "FP.State"=w275:T5)
            n112 = Not Equal?(x=w275, y=w273) -> (x != y?=w274:bool)
            n113 = case shown="True" w274 {
              tunnel: [w284 w286] -> w280
              tunnel: w277 -> [w283 w286]
              tunnel: w276 -> [w282 _]
              tunnel: w273 -> [w281 _]
              frame True {
                n114 = invoke class="VI" method="FP.Open"(reference=w282, error in=w283, "Activate"=TRUE, "State"=w281) -> (error out=w284:errorcluster)  [unwired: 1 in, 4 out]
              }
              frame False {
              }
            }
          }
          frame "Close", "Closed" {
            n115 = property class="VI"(reference=w291, error in=w293) -> (reference out=w290:refnum<vi>, error out=w292:errorcluster, "FP.State"=w288:T5)
            n116 = Not Equal?(x=w288, y=T5."Closed" ("Front Panel Window:State")) -> (x != y?=w287:bool)
            n117 = case shown="True" w287 {
              tunnel: [w295 w298] -> w294
              tunnel: w292 -> [w295 w297]
              tunnel: w290 -> [_ w296]
              frame False {
              }
              frame True {
                n118 = invoke class="VI" method="FP.Close"(reference=w296, error in=w297) -> (error out=w298:errorcluster)  [unwired: 1 in, 2 out]
              }
            }
          }
          frame "Hidden", "Hide" {
            w299 = T5."Hidden" ("State")
            n119 = property class="VI"(reference=w305, error in=w304) -> (reference out=w302:refnum<vi>, error out=w303:errorcluster, "FP.State"=w301:T5)
            n120 = Not Equal?(x=w301, y=w299) -> (x != y?=w300:bool)
            n121 = case shown="True" w300 {
              tunnel: [w310 w311] -> w306
              tunnel: w303 -> [w309 w311]
              tunnel: w302 -> [w308 _]
              tunnel: w299 -> [w307 _]
              frame True {
                n122 = invoke class="VI" method="FP.Open"(reference=w308, error in=w309, "State"=w307) -> (error out=w310:errorcluster)  [unwired: 2 in, 4 out]
              }
              frame False {
              }
            }
          }
          frame "Minimize", "Minimized" {
            w312 = T5."Minimized" ("State")
            n123 = property class="VI"(reference=w318, error in=w317) -> (reference out=w315:refnum<vi>, error out=w316:errorcluster, "FP.State"=w314:T5)
            n124 = Not Equal?(x=w314, y=w312) -> (x != y?=w313:bool)
            n125 = case shown="True" w313 {
              tunnel: [w323 w324] -> w319
              tunnel: w316 -> [w322 w324]
              tunnel: w315 -> [w321 _]
              tunnel: w312 -> [w320 _]
              frame True {
                n126 = invoke class="VI" method="FP.Open"(reference=w321, error in=w322, "State"=w320) -> (error out=w323:errorcluster)  [unwired: 2 in, 4 out]
              }
              frame False {
              }
            }
          }
          frame "Maximize", "Maximized" {
            w325 = T5."Maximized" ("State")
            n127 = property class="VI"(reference=w331, error in=w330) -> (reference out=w328:refnum<vi>, error out=w329:errorcluster, "FP.State"=w327:T5)
            n128 = Not Equal?(x=w327, y=w325) -> (x != y?=w326:bool)
            n129 = case shown="True" w326 {
              tunnel: [w336 w337] -> w332
              tunnel: w329 -> [w335 w337]
              tunnel: w328 -> [w334 _]
              tunnel: w325 -> [w333 _]
              frame True {
                n130 = invoke class="VI" method="FP.Open"(reference=w334, error in=w335, "State"=w333) -> (error out=w336:errorcluster)  [unwired: 2 in, 4 out]
              }
              frame False {
              }
            }
          }
        }
        n131 = call <vilib>:"Add State(s) to Queue__jki_lib_state_machine.vi"("State(s) in (\"\")"=w272) -> ("States Out"=w271:string)  [unwired: 14 in]
      }
      frame "---------- Macro ----------" {
        # "Do not put any code in this frame.\n(It is a separator no-op. You can make a copy of this frame to create a new Macro frame)"
        n132 = call <vilib>:"Add State(s) to Queue__jki_lib_state_machine.vi"("State(s) in (\"\")"=w341) -> ("States Out"=w340:string)  [unwired: 14 in]
      }
      frame "Macro: Initialize" {
        # "Initialization Macro\n(This is called once, when the VI starts)"
        n133 = call <vilib>:"Add State(s) to Queue__jki_lib_state_machine.vi"("State(s) in Front (\"\")"="Data: Initialize\nData: Initialize Graph References\nInitialize Core Data\nUI: Initialize\nUI: Front Panel State >> Open", "State(s) in (\"\")"=w346) -> ("States Out"=w345:string)  [unwired: 13 in]
      }
      frame "Macro: Upload from Local Tree" {
        # "#TODO: Add more checks to make sure only expt folders are selected..."
        # "Initialization Macro\n(This is called once, when the VI starts)"
        n134 = Unbundle By Name(w352) -> ("selected.local path"=w351:path)
        n135 = call-poly <userlib>:"File Exists__ogtk.vi"("file path"=w351) -> ("is directory"=w348:bool, "exists"=w350:bool)  [unwired: 6 in]
        n136 = And(x=w348, y=w350) -> (x .and. y?=w349:bool)
        n137 = case shown="True" w349 {
          tunnel: [" " w359] -> w354
          tunnel: "View before uploading?" -> [_ w358]
          frame False {
            n138 = call "Display Message to User2"() -> ()  [unwired: 10 in, 2 out]
          }
          frame True {
            n139 = case shown="False" w358 {
              tunnel: "Convert: Convert Selected Folder\nLoad: Load Generated TDMS\nProcess: Slice to XY data\nMacro: Visualize\n" -> [w363 w364]
              tunnel: [w362 w364] -> w359
              frame False {
                n140 = call <vilib>:"Add State(s) to Queue__jki_lib_state_machine.vi"("State(s) in (\"\")"=w363, "State(s) at Back (\"\")"="Macro: Upload to AWS" ("State(s) at Back (\"\")")) -> ("States Out"=w362:string)  [unwired: 13 in]
              }
              frame True {
                # "wait to upload file"
              }
            }
          }
        }
        n141 = call <vilib>:"Add State(s) to Queue__jki_lib_state_machine.vi"("State(s) in Front (\"\")"=w354, "State(s) in (\"\")"=w356) -> ("States Out"=w355:string)  [unwired: 13 in]
      }
      frame "Macro: Populate Remote Tree" {
        # "#TODO: should make sure AWS is configured etc. instead of crashing"
        # "Initialization Macro\n(This is called once, when the VI starts)"
        n142 = call <vilib>:"Add State(s) to Queue__jki_lib_state_machine.vi"("State(s) in Front (\"\")"="AWS: Populate Remote Tree", "State(s) in (\"\")"=w369) -> ("States Out"=w368:string)  [unwired: 13 in]
      }
      frame "Macro: Populate Local Tree" {
        # "#TODO: should make sure path is valid or something"
        # "Initialization Macro\n(This is called once, when the VI starts)"
        n143 = call <vilib>:"Add State(s) to Queue__jki_lib_state_machine.vi"("State(s) in Front (\"\")"="Load: Populate Local Tree", "State(s) in (\"\")"=w374) -> ("States Out"=w373:string)  [unwired: 13 in]
      }
      frame "Macro: Visualize" {
        # "#TODO: should rename this macro,\nit only needs to be sliced after the slicing indices are changed"
        n144 = call <vilib>:"Add State(s) to Queue__jki_lib_state_machine.vi"("State(s) in Front (\"\")"="Visualize: Plot Live XY to Intensity\nVisualize: Calculate Histogram\nVisualize: Update Z from Histogram\nVisualize: Line Cuts", "State(s) in (\"\")"=w379) -> ("States Out"=w378:string)  [unwired: 13 in]
      }
      frame "Macro: Upload to AWS" {
        # "#TODO: should rename this macro,\nit only needs to be sliced after the slicing indices are changed"
        # "Initialization Macro\n(This is called once, when the VI starts)"
        n145 = call <vilib>:"Add State(s) to Queue__jki_lib_state_machine.vi"("State(s) in Front (\"\")"="AWS: Upload file\n//AWS: Check if file exists\nAWS: Populate Remote Tree", "State(s) in (\"\")"=w384) -> ("States Out"=w383:string)  [unwired: 13 in]
      }
      frame "Macro: Download from AWS" {
        # "#TODO: should rename this macro,\nit only needs to be sliced after the slicing indices are changed"
        # "Initialization Macro\n(This is called once, when the VI starts)"
        n146 = call <vilib>:"Add State(s) to Queue__jki_lib_state_machine.vi"("State(s) in Front (\"\")"="//AWS: Check if file exists\nAWS: Download file", "State(s) in (\"\")"=w389) -> ("States Out"=w388:string)  [unwired: 13 in]
      }
      frame "Macro: Reslice and perform all ops" {
        # "#TODO: should rename this macro,\nit only needs to be sliced after the slicing indices are changed"
        # "Initialization Macro\n(This is called once, when the VI starts)"
        n147 = call <vilib>:"Add State(s) to Queue__jki_lib_state_machine.vi"("State(s) in Front (\"\")"="Process: Slice to XY data\nProcess: Perform All Operations\nMacro: Visualize", "State(s) in (\"\")"=w394) -> ("States Out"=w393:string)  [unwired: 13 in]
      }
      frame "Macro: Exit" {
        # "Exit Macro\n(This is called once, when the VI exits)"
        n148 = Unbundle By Name(w401) -> ("Core.Close Panel on Exit?"=w400:bool)
        n149 = Select(t="UI: Front Panel State >> Close", s=w400, f="") -> (s? t:f=w397:string)
        n150 = call <vilib>:"Add State(s) to Queue__jki_lib_state_machine.vi"("State(s) in (\"\")"=w397, "State(s) at Back (\"\")"="Data: Cleanup\nExit") -> ("States Out"=w395:string)  [unwired: 13 in]
        n151 = call <vilib>:"Add State(s) to Queue__jki_lib_state_machine.vi"("State(s) in Front (\"\")"=w395, "State(s) in (\"\")"=w404) -> ("States Out"=w403:string)  [unwired: 13 in]
      }
      frame "---------- New Category ----------" {
        # "Template Separator\n(You can make a copy of, or modify, this frame)"
        n152 = call <vilib>:"Add State(s) to Queue__jki_lib_state_machine.vi"("State(s) in (\"\")"=w408) -> ("States Out"=w407:string)  [unwired: 14 in]
      }
      frame "New Category: 1" {
        # "Your code here.\n(You can make a copy of, or modify, this frame)"
        n153 = call <vilib>:"Add State(s) to Queue__jki_lib_state_machine.vi"("State(s) in (\"\")"=w412) -> ("States Out"=w411:string)  [unwired: 14 in]
      }
      frame "New Category: 2" {
        # "Your code here.\n(You can make a copy of, or modify, this frame)"
        n154 = call <vilib>:"Add State(s) to Queue__jki_lib_state_machine.vi"("State(s) in (\"\")"=w416) -> ("States Out"=w415:string)  [unwired: 14 in]
      }
      frame "---------- AWS ----------" {
        # "Template Separator\n(You can make a copy of, or modify, this frame)"
        n155 = call <vilib>:"Add State(s) to Queue__jki_lib_state_machine.vi"("State(s) in (\"\")"=w420) -> ("States Out"=w419:string)  [unwired: 14 in]
      }
      frame "AWS: Check if file exists" {
        # "DEPRECATED"
        # "Your code here.\n(You can make a copy of, or modify, this frame)"
        n156 = Unbundle By Name(w422) -> ()  [unwired: 2 out]
        n157 = call <vilib>:"Add State(s) to Queue__jki_lib_state_machine.vi"("State(s) in (\"\")"=w424) -> ("States Out"=w423:string)  [unwired: 14 in]
      }
      frame "AWS: Populate Remote Tree" {
        # "Your code here.\n(You can make a copy of, or modify, this frame)"
        n158 = Unbundle By Name(w427) -> ("Data.S3"=w431:refnum<class "Data.S3.lvclass">)  [unwired: 1 out]
        n159 = control-ref of="Remote Tree"() -> (w430:refnum<vi>)
        n160 = call <userlib>:"Populate Tree Ctl from Bucket.vi"("error in (no error)"=w429, "Tree Ctl Ref"=w430, "Data.S3"=w431) -> ("error out"=w428:errorcluster, "Data.S3 out"=w425:refnum<class "Data.S3.lvclass">)  [unwired: 4 in, 3 out]
        n161 = Bundle By Name(cluster=w427, "Data.S3"=w425) -> (w426:T11)
        n162 = call <vilib>:"Add State(s) to Queue__jki_lib_state_machine.vi"("State(s) in (\"\")"=w433) -> ("States Out"=w432:string)  [unwired: 14 in]
      }
      frame "AWS: Upload file" {
        w442 = "/"
        # "PPMS2"
        # "reformat name"
        # "SA030.."
        # "031_.."
        # "#TODO: put these values in the\nstate wire..."
        # "Template Separator\n(You can make a copy of, or modify, this frame)"
        n163 = control-ref of="Uploading Indicator"() -> (w448:refnum<vi>)
        n164 = property on="Property Node" class="Bool (strict)"(reference=w448, error in=w450, "Value"=TRUE ("Downloading Indicator")) -> (reference out=w447:refnum<vi>, error out=w440:errorcluster)
        n165 = Unbundle By Name(w456) -> ("generated tdms"=w454:path, "Data.S3"=w458:refnum<class "Data.S3.lvclass">)
        n166 = Strip Path(path=w454) -> (stripped path=w464:path, name=w463:string)
        n167 = Strip Path(path=w464) -> (stripped path=w446:path, name=w461:string)
        n168 = call <userlib>:"Tick Count (ms)__ogtk.vi"("error in (no error)"=w440) -> ("error out"=w439:errorcluster, "millisecond timer value"=w435:u32)  [unwired: 9 in]
        n169 = Strip Path(path=w446) -> (name=w445:string)  [unwired: 1 out]
        n170 = call "replace_bad_aws_characters.vi"("error in (no error)"=w439, "name"=w463) -> ("error out"=w459:errorcluster, "result string"=w462:string)  [unwired: 8 in]
        n171 = call "replace_bad_aws_characters.vi"("error in (no error)"=w459, "name"=w461) -> ("error out"=w444:errorcluster, "result string"=w460:string)  [unwired: 8 in]
        n172 = call "replace_bad_aws_characters.vi"("error in (no error)"=w444, "name"=w445) -> ("error out"=w443:errorcluster, "result string"=w441:string)  [unwired: 8 in]
        n173 = call-poly <userlib>:"File Exists__ogtk.vi"("file path"=w454) -> ("exists"=w465:bool)  [unwired: 6 in, 1 out]
        n174 = Concatenate Strings(w442, w441, w442, w460, w442, w462) -> (w453:string)
        n175 = case shown="True" w465 {
          tunnel: w454 -> [_ w472]
          tunnel: w453 -> [_ w475]
          tunnel: w443 -> [w469 w474]
          tunnel: [w469 w473] -> w438
          tunnel: w458 -> [w468 w471]
          tunnel: [w468 w470] -> w455
          frame False {
            n176 = call "Display Message to User"() -> ()  [unwired: 10 in, 2 out]
          }
          frame True {
            n177 = call <userlib>:"Upload File.vi"("error in (no error)"=w474, "Object Path (including file name)"=w475, "file to upload"=w472, "Data.S3"=w471) -> ("error out"=w473:errorcluster, "Data.S3"=w470:refnum<class "Data.S3.lvclass">)  [unwired: 6 in]
          }
        }
        n178 = call <userlib>:"Tick Count (ms)__ogtk.vi"("error in (no error)"=w438) -> ("error out"=w437:errorcluster, "millisecond timer value"=w436:u32)  [unwired: 9 in]
        n179 = property on="Property Node" class="Bool (strict)"(reference=w447, error in=w437, "Value"=FALSE ("Downloading Indicator")) -> (error out=w449:errorcluster)  [unwired: 1 out]
        n180 = Subtract(x=w436, y=w435) -> (x-y=→"S3 upload (ms)":u32)
        n181 = Bundle By Name(cluster=w456, "Data.S3"=w455, "uploaded remote path"=w453) -> (w457:T11)
        n182 = call <vilib>:"Add State(s) to Queue__jki_lib_state_machine.vi"("State(s) in (\"\")"=w467) -> ("States Out"=w466:string)  [unwired: 14 in]
      }
      frame "AWS: Download file" {
        # "DEPRECATED"
        # "Template Separator\n(You can make a copy of, or modify, this frame)"
        n183 = Unbundle By Name(w486) -> ("local data directory"=w483:path, "Data.S3"=w481:refnum<class "Data.S3.lvclass">)
        n184 = Path To String(path=w483) -> (string=w479:string)
        n185 = call "replace_bad_aws_characters.vi"("error in (no error)"=w477, "name"=w479) -> ("error out"=w476:errorcluster, "result string"=w478:string)  [unwired: 8 in]
        n186 = Concatenate Strings(w478, ".tdms") -> (w484:string)
        n187 = String To Path(string=w484) -> (path=w480:path)
        n188 = call <userlib>:"Download File.vi"("error in (no error)"=w476, "path to store downloaded file"=w480, "Data.S3"=w481) -> ("error out"=w482:errorcluster)  [unwired: 6 in, 2 out]
        n189 = call <vilib>:"Add State(s) to Queue__jki_lib_state_machine.vi"("State(s) in (\"\")"=w488) -> ("States Out"=w487:string)  [unwired: 14 in]
      }
      frame "---------- PostgreSQL ----------" {
        # "Template Separator\n(You can make a copy of, or modify, this frame)"
        n190 = call <vilib>:"Add State(s) to Queue__jki_lib_state_machine.vi"("State(s) in (\"\")"=w492) -> ("States Out"=w491:string)  [unwired: 14 in]
      }
      frame "PostgreSQL: Configure Connection" {
        # "Template Separator\n(You can make a copy of, or modify, this frame)"
        n191 = Unbundle By Name(w494) -> ("Data.PG in"=w493:refnum<class "Data.PGSQL.lvclass">)
        n192 = call <userlib>:"Set Connection Info.vi"("Data.PG in"=w493) -> ()  [unwired: 8 in, 2 out]
        n193 = call <vilib>:"Add State(s) to Queue__jki_lib_state_machine.vi"("State(s) in (\"\")"=w497) -> ("States Out"=w496:string)  [unwired: 14 in]
      }
      frame "PostgreSQL: Upload Data" {
        # "Template Separator\n(You can make a copy of, or modify, this frame)"
        n194 = call <vilib>:"Add State(s) to Queue__jki_lib_state_machine.vi"("State(s) in (\"\")"=w501) -> ("States Out"=w500:string)  [unwired: 14 in]
      }
      frame "---------- Process ----------" {
        # "Template Separator\n(You can make a copy of, or modify, this frame)"
        n195 = call <vilib>:"Add State(s) to Queue__jki_lib_state_machine.vi"("State(s) in (\"\")"=w505) -> ("States Out"=w504:string)  [unwired: 14 in]
      }
      frame "Process: Slice to XY data" {
        # "#TODO: add ring ctls for channels\n(tdms has a function for this)"
        # "no operations performed\nyet on freshly sliced data"
        # "have 3D array (pages of 2D arrays containing channels vs time)"
        # "Template Separator\n(You can make a copy of, or modify, this frame)"
        n196 = call <userlib>:"Tick Count (ms)__ogtk.vi"("error in (no error)"=w530) -> ("error out"=w518:errorcluster, "millisecond timer value"=w527:u32)  [unwired: 9 in]
        n197 = Unbundle By Name(w525) -> ("Data Save"=w520:refnum<class "Data.lvclass">, "data dimensions"=w508:i32[])
        n198 = Index Array(array=w508, index=0) -> (element=w506:i32)
        n199 = property on="updating" class="Bool (strict)"(error in=w518, "Value"=TRUE ("updating")) -> ()  [unwired: 1 in, 2 out]
        n200 = call <userlib>:"Read Data (Dictionary).vi"("error in (no error)"=w518, "Data Save"=w520) -> ("error out"=w517:errorcluster, "Data (Dictionary)"=w514:T15[], "Data Save out"=w519:refnum<class "Data.lvclass">)  [unwired: 7 in]
        n201 = call <userlib>:"Read Wavenames.vi"("error in (no error)"=w517, "Data Save"=w519) -> ("error out"=w510:errorcluster, "Wavenames"=→"Wavenames":string[], "Data Save out"=w516:refnum<class "Data.lvclass">)  [unwired: 7 in]
        n202 = call "Data(dictionary) to XY.vi"("dimension size (hmm)"=w506, "error in (no error)"=w510, "IV Y wavename"="AI4", "IV X wavename"="AO3", "Data (Dictionary)"=w514) -> ("error out"=w509:errorcluster, "wacky arary"=w513:cluster{dbl[], dbl[]}[])  [unwired: 5 in]
        n203 = Bundle By Name(cluster=w525, "active XY data"=w513, "operations performed"=string[] [], "Data Save"=w516) -> (w524:T11)
        n204 = call <userlib>:"Tick Count (ms)__ogtk.vi"("error in (no error)"=w509) -> ("error out"=w529:errorcluster, "millisecond timer value"=w528:u32)  [unwired: 9 in]
        n205 = Subtract(x=w528, y=w527) -> (x-y=→"slicing\ntime":u32)
      }
      frame "Process: Check for Updates" {
        # "'no need'"
        # "if these are NOT equal\nthen it needs to be resliced\n-> result must be false"
        # "tru if all match"
        # "have 3D array (pages of 2D arrays containing channels vs time)"
        # "Template Separator\n(You can make a copy of, or modify, this frame)"
        n206 = Unbundle By Name(w543) -> ("operations performed"=w539:string[], "Operations List"=w544:refnum<vi>)
        n207 = Array Size(array=w539) -> (size(s)=w537:i32)
        n208 = property on="Property Node" class="LstBox (strict)"(reference=w544) -> ("Item Names"=w538:string[])  [unwired: 1 in, 2 out]
        n209 = Array Size(array=w538) -> (size(s)=w536:i32)
        n210 = Not Equal?(x=w537, y=w536) -> (x != y?=w533:bool)
        n211 = Equal?(x=w539, y=w538) -> (x = y?=w535:bool[])
        n212 = And Array Elements(Boolean array=w535) -> (logical AND=w532:bool)
        n213 = Not(x=w532) -> (.not. x?=w531:bool)
        n214 = Or(x=w531, y=w533) -> (x .or. y?=w534:bool)
        n215 = case shown="True" w534 {
          tunnel: ["" "Macro: Reslice and perform all ops"] -> w540
          frame False {
          }
          frame True {
            # "if the performed operations\ndon't match the desired list\nthen data needs updated 0_0"
          }
        }
        n216 = call <vilib>:"Add State(s) to Queue__jki_lib_state_machine.vi"("State(s) in Front (\"\")"=w540, "State(s) in (\"\")"=w542) -> ("States Out"=w541:string)  [unwired: 13 in]
      }
      frame "Process: Add Operation" {
        # "#OPERATIONS"
        # "have 3D array (pages of 2D arrays containing channels vs time)"
        # "Template Separator\n(You can make a copy of, or modify, this frame)"
        n217 = Unbundle By Name(w555) -> ("Operations List"=w554:refnum<vi>)
        n218 = Unbundle By Name(w555) -> ("dictionary out"=w556:T10)
        n219 = case shown="\"fft\"" "Operation Config" {
          tunnel: [w560 "fft"] -> w559
          tunnel: w556 -> [w563 w567]
          tunnel: w558 -> [w562 w569]
          tunnel: [w561 w568] -> w557
          frame "derivative", Default {
            # "key = stringified derivative\nvalue = the derivative parameter cluster"
            n220 = call "derivative_toString.vi"("derivative"="derivative") -> ("concatenated string"=w560:string)  [unwired: 10 in]
            n221 = Bundle("concatenated string"=w560, "derivative"="derivative") -> (w565:T16)  [unwired: 1 in]
            n222 = call-poly <userlib>:"Dictionary Update__ogtk.vi"("error in (no error)"=w562, "key-value"=w565, "dictionary"=w563) -> ("error out"=w561:errorcluster)  [unwired: 6 in, 2 out]
          }
          frame "fft" {
            n223 = Bundle("fft", "fft"=T7 {"fft"="fft"}) -> (w571:cluster{string, "fft":T7})  [unwired: 1 in]
            n224 = call-poly <userlib>:"Dictionary Update__ogtk.vi"("error in (no error)"=w569, "key-value"=w571, "dictionary"=w567) -> ("error out"=w568:errorcluster)  [unwired: 6 in, 2 out]
          }
        }
        n225 = property on="Property Node" class="LstBox (strict)"(reference=w554) -> (reference out=w551:refnum<vi>, "Item Names"=w553:string[])  [unwired: 1 in, 1 out]
        n226 = Build Array (concatenate)(w553, w559) -> (w552:string[])
        n227 = property on="Property Node" class="LstBox (strict)"(reference=w551, "Item Names"=w552, "Val(Sgnl)"=0 ("Value (Signaling)")) -> ()  [unwired: 1 in, 2 out]
      }
      frame "Process: Perform All Operations" {
        # "dict keys are \nunique operation \nidentifier strings"
        # "have 3D array (pages of 2D arrays containing channels vs time)"
        # "Template Separator\n(You can make a copy of, or modify, this frame)"
        n228 = Unbundle By Name(w579) -> ("dictionary out"=w575:T10, "Operations List"=w581:refnum<vi>)
        n229 = property on="Property Node" class="LstBox (strict)"(reference=w581) -> ("Item Names"=w573:string[])  [unwired: 1 in, 2 out]
        n230 = Unbundle By Name(w579) -> ("active XY data"=w577:T13)
        n231 = for {
          tunnel: w573 -> [w593] mode=indexing
          shift-right: [w592] -> _
          shift-left: w575 -> [w582]
          shift-right: [w584] -> _
          shift-left: _ -> [w589]
          shift-right: [w586] -> w574
          shift-left: w577 -> [w587]
          tunnel: [w583] -> _ mode=indexing
          # "the label of the first cluster element must describe the operation"
          # "#OPERATIONS"
          n232 = call <userlib>:"Dictionary Get Value__ogtk.vi"("error in"=w589, "key"=w593, "dictionary"=w582) -> ("error out"=w590:errorcluster, "value"=w588:variant, "dictionary out"=w592:T10)  [unwired: 5 in, 1 out]
          n233 = call <userlib>:"Get Cluster Element Names__ogtk.vi"("error in (no error)"=w590, "Cluster"=w588) -> ("error out"=w585:errorcluster, "Element Names"=w591:string[])  [unwired: 8 in]
          n234 = Index Array(array=w591) -> (element=w583:string)  [unwired: 1 in]
          n235 = case shown="\"fft\", Default" w583 {
            tunnel: w588 -> [_ w608]
            tunnel: w587 -> [w599 w606]
            tunnel: [w595 w605] -> w586
            tunnel: w585 -> [w598 w607]
            tunnel: [w596 w604] -> w584
            frame "fft", Default {
              n236 = call <userlib>:"FFT (multiple).vi"("error in (no error)"=w598, "XY-data"=w599) -> ("error out"=w597:errorcluster, "magnitude []"=w594:cluster{"f0":dbl, "df":dbl, "magnitude":dbl[]}[])  [unwired: 6 in, 2 out]
              n237 = call "freq_magnitude_to_XY.vi"("error in (no error)"=w597, "magnitude []"=w594) -> ("error out"=w596:errorcluster, "freq_magnitude_XY"=w595:cluster{dbl[], "magnitude":dbl[]}[])  [unwired: 8 in]
            }
            frame "derivative" {
              n238 = Variant To Data(type=T8 {"derivative"="derivative", "Interval"=2.0, "Interval Units"=enum."Points", "Type"=enum."dy/dx vs x"} ("derivative"), Variant=w608) -> (data=w609:T8)  [unwired: 1 in, 1 out]
              n239 = Unbundle By Name(w609) -> ("Interval"=w603:dbl, "Interval Units"=w601:enum16{"Points", "Data"}, "Type"=w602:enum16{"dy/dx vs x", "dx/dy vs y"})
              n240 = call-poly <userlib>:"Derivative.vi"("Interval Units"=w601, "error in (no error)"=w607, "Type"=w602, "Interval"=w603, "XY-data"=w606) -> ("error out"=w604:errorcluster, "Differential out"=w605:cluster{"X-array":dbl[], "Y-array":dbl[]}[])  [unwired: 4 in, 1 out]
            }
          }
        }
        n241 = Bundle By Name(cluster=w579, "active XY data"=w574, "operations performed"=w573) -> (w578:T11)
      }
      frame "---------- Visualize ----------" {
        # "Template Separator\n(You can make a copy of, or modify, this frame)"
        n242 = call <vilib>:"Add State(s) to Queue__jki_lib_state_machine.vi"("State(s) in (\"\")"=w613) -> ("States Out"=w612:string)  [unwired: 14 in]
      }
      frame "Visualize: Plot Live XY to Intensity" {
        # "#TODO: Shouldnt go in here"
        n243 = Unbundle By Name(w621) -> ("graphs"=w625:refnum<class "graph_utilities.lvclass">[], "active XY data"=w624:T13)
        n244 = call "XYs_to_Intensity.vi"("error in (no error)"=w622, "XYs in"=w624) -> ("error out"=w623:errorcluster, "Intensity data (y) out"=w626:dbl[][])  [unwired: 8 in]
        n245 = Index Array(array=w625) -> (element=w627:refnum<class "graph_utilities.lvclass">)  [unwired: 1 in]
        n246 = call <userlib>:"Set Intensity Graph Value.vi"("error in (no error)"=w623, "Value"=w626, "graph_utilities in"=w627) -> ("error out"=w616:errorcluster, "graph_utilities out"=w617:refnum<class "graph_utilities.lvclass">)  [unwired: 7 in]
        n247 = call <userlib>:"Set Intensity Graph Z Color.vi"("error in (no error)"=w616, "Colors []"=u32[] [10420479, 16860, 3381759, 6618880, 16772608, 16711680], "graph_utilities in"=w617) -> ("error out"=w615:errorcluster)  [unwired: 7 in, 1 out]
        n248 = property on="updating" class="Bool (strict)"(error in=w615, "Value"=FALSE ("updating")) -> (error out=w620:errorcluster)  [unwired: 1 in, 1 out]
        n249 = call <vilib>:"Add State(s) to Queue__jki_lib_state_machine.vi"("State(s) in Front (\"\")"="Visualize: Calculate Histogram" ("State(s) in Front (\"\")"), "State(s) in (\"\")"=w629) -> ("States Out"=w628:string)  [unwired: 13 in]
      }
      frame "Visualize: Calculate Histogram" {
        n250 = Unbundle By Name(w640) -> ("Histogram Graph"=w636:refnum<vi>, "active XY data"=w642:T13)
        n251 = call "XYs_to_Intensity.vi"("error in (no error)"=w641, "XYs in"=w642) -> ("error out"=w638:errorcluster, "Intensity data (y) out"=w639:dbl[][])  [unwired: 8 in]
        n252 = call "calculate_histogram.vi"("error in (no error)"=w638, "# std deviations for histogram width (1)"="# std deviations for\nhistogram width", "2D arr Intensity Graph"=w639) -> ("error out"=w635:errorcluster, "Histogram Graph"=w637:T1)  [unwired: 5 in, 2 out]
        n253 = property class="XYGraph (strict)"(reference=w636, error in=w635, "Value"=w637) -> (reference out=w634:refnum<vi>, error out=w633:errorcluster)
        n254 = call "adjust_histogram_cursor.vi"("error in (no error)"=w633, "lock to bin edges"=TRUE, "histogram reference"=w634) -> ("error out"=w632:errorcluster)  [unwired: 8 in]
        n255 = call <vilib>:"Add State(s) to Queue__jki_lib_state_machine.vi"("State(s) in (\"\")"=w644) -> ("States Out"=w643:string)  [unwired: 14 in]
      }
      frame "Visualize: Update Z from Histogram" {
        # "#TODO: adjust line cut scales\nhere also"
        n256 = Unbundle By Name(w660) -> ("graphs"=w656:refnum<class "graph_utilities.lvclass">[], "Histogram Graph"=w657:refnum<vi>)
        n257 = property on="Property Node" class="XYGraph (strict)"(reference=w657, error in=w654, "Active Cursor"=u32 0, "Active Cursor"=u32 1) -> (error out=w649:errorcluster, "Cursor.Cursor X"=w648:dbl, "Cursor.Cursor X"=w647:dbl)  [unwired: 1 out]
        n258 = control-ref of="Horizontal Linecut"() -> (w646:refnum<vi>)
        n259 = control-ref of="Vertical Linecut"() -> (w645:refnum<vi>)
        n260 = disable-structure shown="Enabled" {
          disable-tunnel: w656 -> [w663 _]
          disable-tunnel: [_ w664] -> w655
          frame Disabled {
            # "Should have a graphutils\nvi for Z range setting here"
            n261 = Index Array(array=w663) -> ()  [unwired: 1 in, 1 out]
          }
          frame Enabled {
            n262 = control-ref of="Intensity Graph"() -> (w664:refnum<vi>)
          }
        }
        n263 = property on="Property Node" class="IntGraph (strict)"(reference=w655, error in=w649, "ZScale.Minimum"=w648, "ZScale.Maximum"=w647) -> (error out=w652:errorcluster)  [unwired: 1 out]
        n264 = property on="Property Node" class="XYGraph (strict)"(reference=w646, error in=w649, "YScale.Minimum"=w648, "YScale.Maximum"=w647) -> (error out=w651:errorcluster)  [unwired: 1 out]
        n265 = property on="Property Node" class="XYGraph (strict)"(reference=w645, error in=w649, "YScale.Minimum"=w648, "YScale.Maximum"=w647) -> (error out=w650:errorcluster)  [unwired: 1 out]
        n266 = Merge Errors(w652, w651, w650) -> (w653:errorcluster)
        n267 = call <vilib>:"Add State(s) to Queue__jki_lib_state_machine.vi"("State(s) in (\"\")"=w662) -> ("States Out"=w661:string)  [unwired: 14 in]
      }
      frame "Visualize: Line Cuts" {
        w665 = 42.0 ("width (vertical)")
        n268 = disable-structure shown="Disabled" {
          frame Disabled {
            n269 = call <userlib>:"Linecut Example.vi"() -> ()  [unwired: 12 in]
          }
          frame Enabled {
          }
        }
        n270 = Unbundle By Name(w674) -> ("graphs"=w671:refnum<class "graph_utilities.lvclass">[])
        n271 = Index Array(array=w671, index #1=1 ("index"), index #2=2 ("index")) -> (element #1=w670:refnum<class "graph_utilities.lvclass">, element #2=w669:refnum<class "graph_utilities.lvclass">)
        n272 = call <userlib>:"Intensity Graph Linecut (Vertical).vi"("error in (no error)"=w667, "width (vertical)"=w665, "graph_utilities in"=w670) -> ("error out"=w668:errorcluster)  [unwired: 7 in, 1 out]
        n273 = call <userlib>:"Intensity Graph Linecut (Horizontal).vi"("error in (no error)"=w668, "width (horizontal)"=w665, "graph_utilities in"=w669) -> ("error out"=w666:errorcluster)  [unwired: 7 in, 1 out]
        n274 = call <vilib>:"Add State(s) to Queue__jki_lib_state_machine.vi"("State(s) in (\"\")"=w676) -> ("States Out"=w675:string)  [unwired: 14 in]
      }
      frame "---------- Load ----------" {
        # "Template Separator\n(You can make a copy of, or modify, this frame)"
        n275 = call <vilib>:"Add State(s) to Queue__jki_lib_state_machine.vi"("State(s) in (\"\")"=w680) -> ("States Out"=w679:string)  [unwired: 14 in]
      }
      frame "Load: Load Generated TDMS" {
        # "#TODO: clean up frame with more subvis\nalso this will get messed up if a 'single data\npoint' channel is the first one..."
        # "Template Separator\n(You can make a copy of, or modify, this frame)"
        n276 = property on="Visualizing Indicator" class="Bool (strict)"(error in=w707, "Value"=TRUE ("read cache")) -> (error out=w698:errorcluster)  [unwired: 1 in, 1 out]
        n277 = Unbundle By Name(w703) -> ("Data Save"=w696:refnum<class "Data.lvclass">, "generated tdms"=w681:path)
        n278 = call <userlib>:"Tick Count (ms)__ogtk.vi"("error in (no error)"=w698) -> ("error out"=w687:errorcluster, "millisecond timer value"=w700:u32)  [unwired: 9 in]
        n279 = call "Read Unparsed Metadata from TDMS.vi"("error in (no error)"=w687, "file path"=w681) -> ("error out"=w685:errorcluster)  [unwired: 7 in, 2 out]
        n280 = call <userlib>:"Data Read.vi"("Append Index"=-1, "error in (no error)"=w685, "path"=w681) -> ("error out"=w693:errorcluster, "Notes"=→"Notes":string, "Data (Dictionary)"=w689:T15[])  [unwired: 5 in, 1 out]
        n281 = call <userlib>:"Write Data (Dictionary).vi"("error in (no error)"=w693, "Data (Dictionary)"=w689, "Data Save"=w696) -> ("error out"=w691:errorcluster, "Data Save out"=w692:refnum<class "Data.lvclass">)  [unwired: 7 in]
        n282 = call <userlib>:"Read Wavenames.vi"("error in (no error)"=w691, "Data Save"=w692) -> ("error out"=w682:errorcluster, "Wavenames"=w695:string[], "Data Save out"=w683:refnum<class "Data.lvclass">)  [unwired: 7 in]
        n283 = call "TDMS Get Number of Groups.vi"("error in (no error)"=w682, "path"=w681) -> ("error out"=w686:errorcluster, "# of groups"=w688:i32)  [unwired: 8 in]
        n284 = call "get data dimensions.vi"("# of groups"=w688, "Data (Dictionary)"=w689) -> ("data dimensions"=w694:i32[])  [unwired: 8 in, 1 out]
        "data dimensions" <- w694
        n285 = call <userlib>:"Tick Count (ms)__ogtk.vi"("error in (no error)"=w686) -> ("error out"=w697:errorcluster, "millisecond timer value"=w701:u32)  [unwired: 9 in]
        n286 = Bundle By Name(cluster=w703, "Data Save"=w683, "wavenames"=w695, "data dimensions"=w694) -> (w702:T11)
        n287 = Subtract(x=w701, y=w700) -> (x-y=→"TDMS load (ms)":u32)
        n288 = property on="Visualizing Indicator" class="Bool (strict)"(error in=w697, "Value"=FALSE ("read cache")) -> (error out=w705:errorcluster)  [unwired: 1 in, 1 out]
        n289 = call <vilib>:"Add State(s) to Queue__jki_lib_state_machine.vi"("State(s) in (\"\")"=w709) -> ("States Out"=w708:string)  [unwired: 14 in]
      }
      frame "Load: Populate Local Tree" {
        # "only show tdms files"
        n290 = Unbundle By Name(w721) -> ("local data directory"=w715:path)
        n291 = List Folder(path=w715, error in=w711) -> (path out=w714:path, folder names=w713:string[], error out=w710:errorcluster)  [unwired: 2 in, 1 out]
        n292 = call-poly <userlib>:"Build Path__ogtk.vi"("name or relative path"=w713, "base path"=w714) -> ("appended path"=w712:path[])
        n293 = control-ref of="Local Tree"() -> (w719:refnum<vi>)
        n294 = invoke class="Tree (strict)" method="Edit Tree Items.Delete"(reference=w719, error in=w710) -> (reference out=w718:refnum<vi>, error out=w716:errorcluster)  [unwired: 3 in, 3 out]
        n295 = Path To String(path=w712) -> (string=w720:string[])
        n296 = for {
          tunnel: w718 -> [w725]
          tunnel: w720 -> [w724] mode=indexing
          shift-right: [w726] -> w717
          shift-left: w716 -> [w727]
          n297 = call "recursively populate local tree ctl.vi"("error in (no error)"=w727, "Object path"=w724, "tree ctl ref"=w725) -> ("error out"=w726:errorcluster)  [unwired: 7 in, 1 out]
        }
        n298 = call <vilib>:"Add State(s) to Queue__jki_lib_state_machine.vi"("State(s) in (\"\")"=w723) -> ("States Out"=w722:string)  [unwired: 14 in]
      }
      frame "---------- Convert ----------" {
        n299 = call <vilib>:"Add State(s) to Queue__jki_lib_state_machine.vi"("State(s) in (\"\")"=w731) -> ("States Out"=w730:string)  [unwired: 14 in]
      }
      frame "Convert: Convert Selected Folder" {
        # "expt folder"
        # "unnecessary now for tdms\nunless we want to store in a different location"
        # "replaceorcreate"
        # "#TODO: 'to generate or not to generate' logic\nshould probably go in a different frame"
        # "if regen cache or not exist:"
        n300 = control-ref of="Converting Indicator"() -> (w739:refnum<vi>)
        n301 = property on="Property Node" class="Bool (strict)"(reference=w739, error in=w742, "Value"=TRUE ("working")) -> (reference out=w738:refnum<vi>, error out=w745:errorcluster)
        n302 = call <userlib>:"Tick Count (ms)__ogtk.vi"("error in (no error)"=w745) -> ("error out"=w736:errorcluster, "millisecond timer value"=w747:u32)  [unwired: 9 in]
        n303 = Unbundle By Name(w734) -> ("selected.local path"=w737:path)
        "selected.local path" <- w737
        n304 = call "TDMS path from Experiment Folder.vi"("error in (no error)"=w736, "experiment folder"=w737) -> ("error out"=w735:errorcluster, "tdms file path"=w732:path)  [unwired: 7 in, 1 out]
        "generated tdms file path" <- w732
        n305 = call <userlib>:"Convert Experiment Folder.vi"("error in (no error)"=w735, "Experiment Folder File Type"=File_Type--enum."ITX", "Experiment Folder Path"=w737) -> ("error out"=w740:errorcluster)  [unwired: 8 in]
        n306 = call "Parse and Attach Metadata to TDMS.vi"("error in (no error)"=w740, "experiment folder"=w737) -> ("error out"=w744:errorcluster)  [unwired: 8 in, 1 out]
        n307 = Bundle By Name(cluster=w734, "generated tdms"=w732) -> (w733:T11)
        n308 = call <userlib>:"Tick Count (ms)__ogtk.vi"("error in (no error)"=w744) -> ("error out"=w743:errorcluster, "millisecond timer value"=w748:u32)  [unwired: 9 in]
        n309 = Subtract(x=w748, y=w747) -> (x-y=→"generate TDMS (ms)":u32)
        n310 = property on="Property Node" class="Bool (strict)"(reference=w738, error in=w743, "Value"=FALSE ("working")) -> ()  [unwired: 2 out]
        n311 = call <vilib>:"Add State(s) to Queue__jki_lib_state_machine.vi"("State(s) in (\"\")"=w752) -> ("States Out"=w751:string)  [unwired: 14 in]
      }
    }
  }
  n312 = disable-structure shown="Disabled" {
    frame Disabled {
    }
    frame Enabled {
    }
  }
